vi "new recipe file.vi"() -> ()   [LabVIEW 2018]
uses:
  <vilib>/Utility/file.llb/Read Delimited Spreadsheet (string).vi
panel:
  out "error out 2":errorcluster caption="error out"
  out "error out":errorcluster
  in  "hidden tab":enum32{"Page 1"}(tab)
  out "L pressure":string
  out "L argon flow":string
  out "L rf length step 10":string
  out "L rf length step 9":string
  out "L rf length step 8":string
  out "L rf length step 7":string
  out "L rf length step 6":string
  out "L rf length step 5":string
  out "L rf length step 4":string
  out "L rf length step 3":string
  out "L rf length step 2":string
  out "L rf length step 1":string
  out "L rf power step 10":string
  out "L rf power step 9":string
  out "L rf power step 8":string
  out "L rf power step 7":string
  out "L rf power step 6":string
  out "L rf power step 5":string
  out "L rf power step 4":string
  out "L rf power step 3":string
  out "L rf power step 2":string
  out "L rf power step 1":string
  out "L dc length step 10":string
  out "L dc length step 9":string
  out "L dc length step 8":string
  out "L dc length step 7":string
  out "L dc length step 6":string
  out "L dc length step 5":string
  out "L dc length step 4":string
  out "L dc length step 3":string
  out "L dc length step 2":string
  out "L dc length step 1":string
  out "L dc power step 10":string
  out "L dc power step 9":string
  out "L dc power step 8":string
  out "L dc power step 7":string
  out "L dc power step 6":string
  out "L dc power step 5":string
  out "L dc power step 4":string
  out "L dc power step 3":string
  out "L dc power step 2":string
  out "L dc power step 1":string
  out "L microwave power":string
  out "L chamber selection":string
  out "L single process type selection":string
  out "L tension  value":string
  out "L web speed":string
  out "L web thickness":string
  out "L left init diamater":string
  out "L core diamater":string
  out "L web selection":string
  out "L recipe selection":string
  out "L sbs name":string
  out "L recipe name":string
  out "total length error":bool
  out "left diameter after roll":dbl=8.0
  out "done":bool
  out "L dc step number":string
  out "L rf step number":string
  in  "steplist tab RF":enum32{"Page 1", "Page 2"}(tab)
  in  "rf step watt 1":dbl
  in  "rf step watt 2":dbl
  in  "rf step watt 3":dbl
  in  "rf step watt 4":dbl
  in  "rf step watt 7":dbl
  in  "rf step watt 8":dbl
  in  "rf step watt 5":dbl
  in  "rf step watt 6":dbl
  in  "rf step watt 9":dbl
  in  "rf step watt 10":dbl
  in  "rf step length 1":dbl
  in  "rf step length 2":dbl
  in  "rf step length 3":dbl
  in  "rf step length 4":dbl
  in  "rf step length 5":dbl
  in  "rf step length 6":dbl
  in  "rf step length 7":dbl
  in  "rf step length 8":dbl
  in  "rf step length 9":dbl
  in  "rf step length 10":dbl
  in  "Step Number RF":u16(ring) items=["step 1"=1, "step 2"=2, "step 3"=3, "step 4"=4, "step 5"=5, "step 6"=6, "step 7"=7, "step 8"=8, "step 9"=9, "step 10"=10]
  out "concatenated string":string
  in  "steplist tab DC":enum32{"Page 1", "Page 2"}(tab)
  in  "dc step watt 1":dbl
  in  "dc step watt 2":dbl
  in  "dc step watt 3":dbl
  in  "dc step watt 4":dbl
  in  "dc step watt 5":dbl
  in  "dc step watt 6":dbl
  in  "dc step watt 7":dbl
  in  "dc step watt 8":dbl
  in  "dc step watt 9":dbl
  in  "dc step watt 10":dbl
  in  "dc step length 1":dbl
  in  "dc step length 2":dbl
  in  "dc step length 3":dbl
  in  "dc step length 4":dbl
  in  "dc step length 5":dbl
  in  "dc step length 6":dbl
  in  "dc step length 7":dbl
  in  "dc step length 8":dbl
  in  "dc step length 9":dbl
  in  "dc step length 10":dbl
  in  "Step Number DC":u16(ring) items=["step 1"=1, "step 2"=2, "step 3"=3, "step 4"=4, "step 5"=5, "step 6"=6, "step 7"=7, "step 8"=8, "step 9"=9, "step 10"=10]
  in  "General tab sub vi":enum32{"Page 1"}(tab)
  in  "Pressure set mbar":dbl=0.005 format="%#_1e"
  in  "Ar set sccm":dbl=20.0
  in  "CANCEL":bool
  in  "SAVE":bool
  in  "web-other tab":T1(tab)
  out "total length":dbl=500.0
  in  "tension value":dbl=7.0
  in  "web speed":dbl=250.0
  in  "web thickness":dbl=50.0
  in  "left initial diameter":dbl=94.0
  in  "core diameter":dbl=93.0
  in  "CALCULATE":bool
  in  "Web Selection":u16(ring) items=["web", "other"]
  in  "Recipe Selection":u16(ring) items=["single recipe", "multilayer recipe"]
  in  "Recipe Name":string
  in  "Substrate Material":string
  in  "recipe selection":T2(tab)
  in  "single process selection":enum32{"microwave", "dcsputter", "rfsputter"}(radio)
  in  "single process selection":T3(tab)
  in  "power microwave":dbl
  in  "DC Sputter Chamber Selection":enum32{"chamber II", "chamber III"}(radio)
  in  "power rf":dbl
  in  "web speed ch III ml":dbl=250.0
  in  "web speed ch II ml":dbl=250.0
  in  "LOAD":bool
  in  "password":bool
  in  "password":string
  # "Step List(RF)"
  # "power(watt)"
  # "length(cm)"
  # "Step 1"
  # "Step 2"
  # "Step 3"
  # "Step 4"
  # "Step 5"
  # "Step 6"
  # "Step 7"
  # "Step 8"
  # "Step 9"
  # "Step 10"
  # "Step List(DC)"
  # "power(watt)"
  # "length(cm)"
  # "Step 1"
  # "Step 2"
  # "Step 3"
  # "Step 4"
  # "Step 5"
  # "Step 6"
  # "Step 7"
  # "Step 8"
  # "Step 9"
  # "Step 10"
  # "Recipe Name"
  # "Subsrate Material"
  # "Recipe Selection"
  # "Web Selection"
  # "Argon Flow"
  # "sccm"
  # "Set Pressure"
  # "mbar"
  # "Core Diameter"
  # "mm"
  # "Web Speed"
  # "cm/min"
  # "Left InitialDiameter"
  # "mm"
  # "Tension Value"
  # "N"
  # "µm"
  # "cm"
  # "Web Thickness"
  # "Total Length"
  # "Power"
  # "watt"
  # "Power"
  # "watt"
  # "DCPS PARAMETERS"
  # "Chamber III"
  # "Chamber II"
  # "Web Speed"
  # "cm/min"
  # "Web Speed"
  # "cm/min"
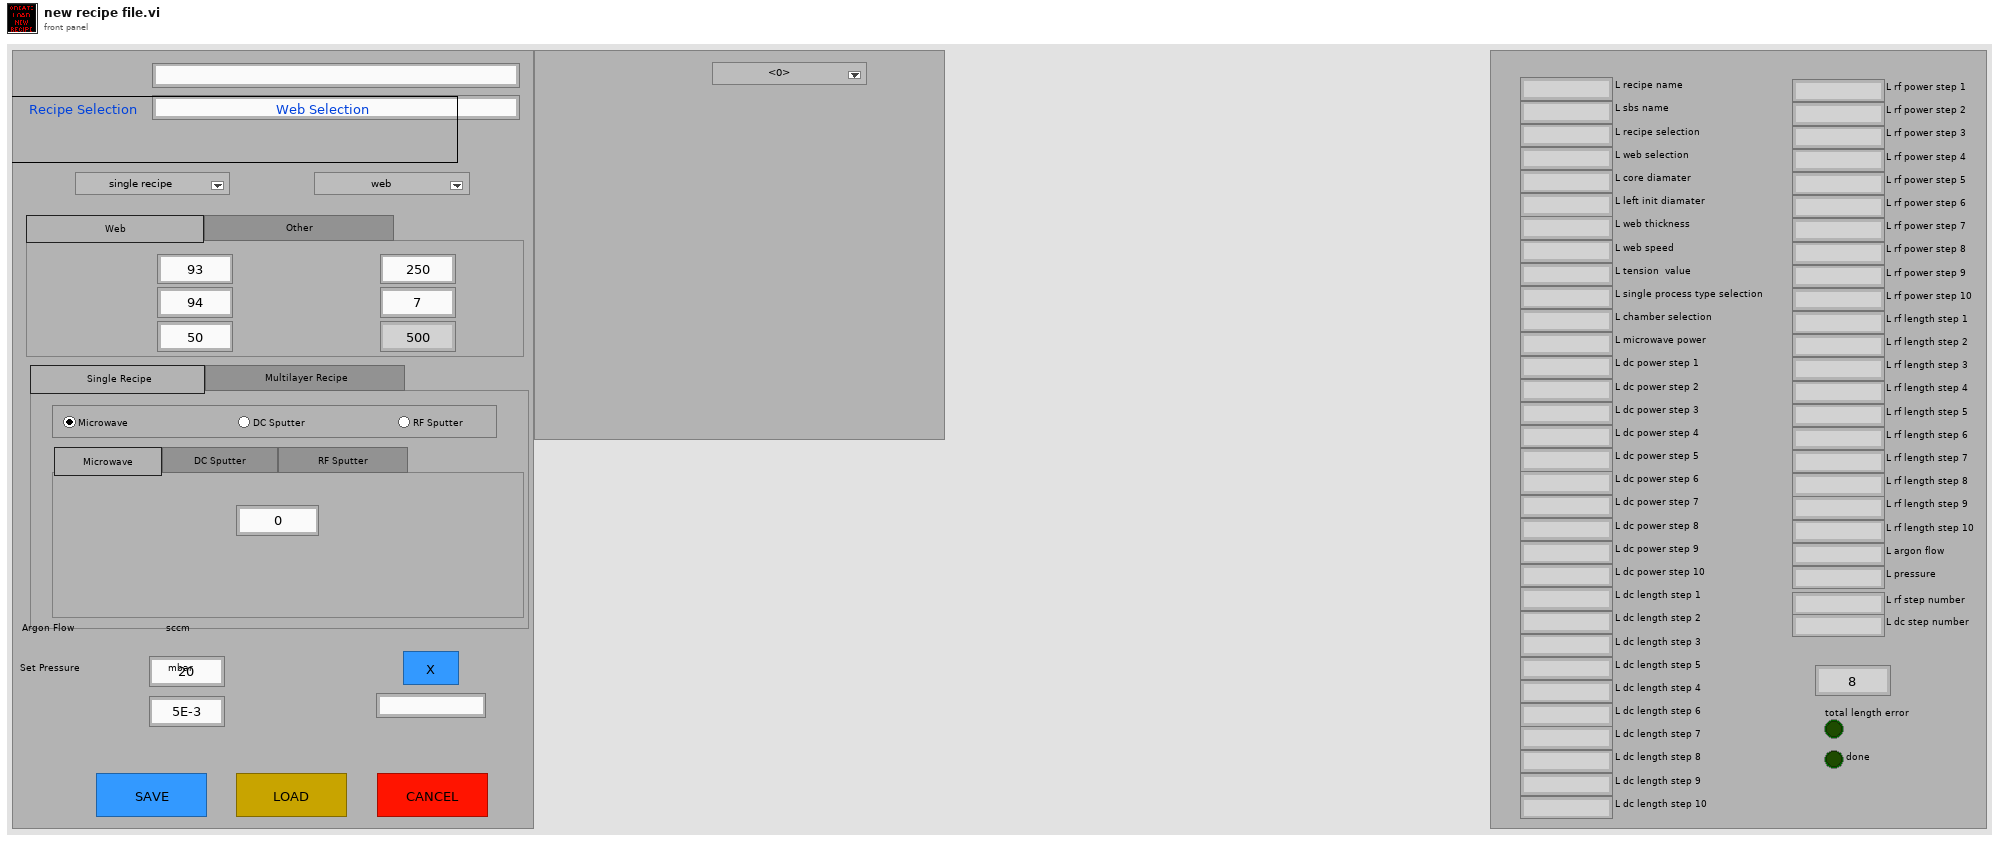
[diagram p1: front panel]
types:
  T1 = enum32{"Web                                                    ", "Other                                                      "}
  T2 = enum32{"Single Recipe                                    ", "Multilayer Recipe                                      "}
  T3 = enum32{"Microwave                ", "DC Sputter                   ", "RF Sputter                         "}
  T4 = enum16{"open", "replace", "create", "open or create", "replace or create", "replace or create with confirmation"}
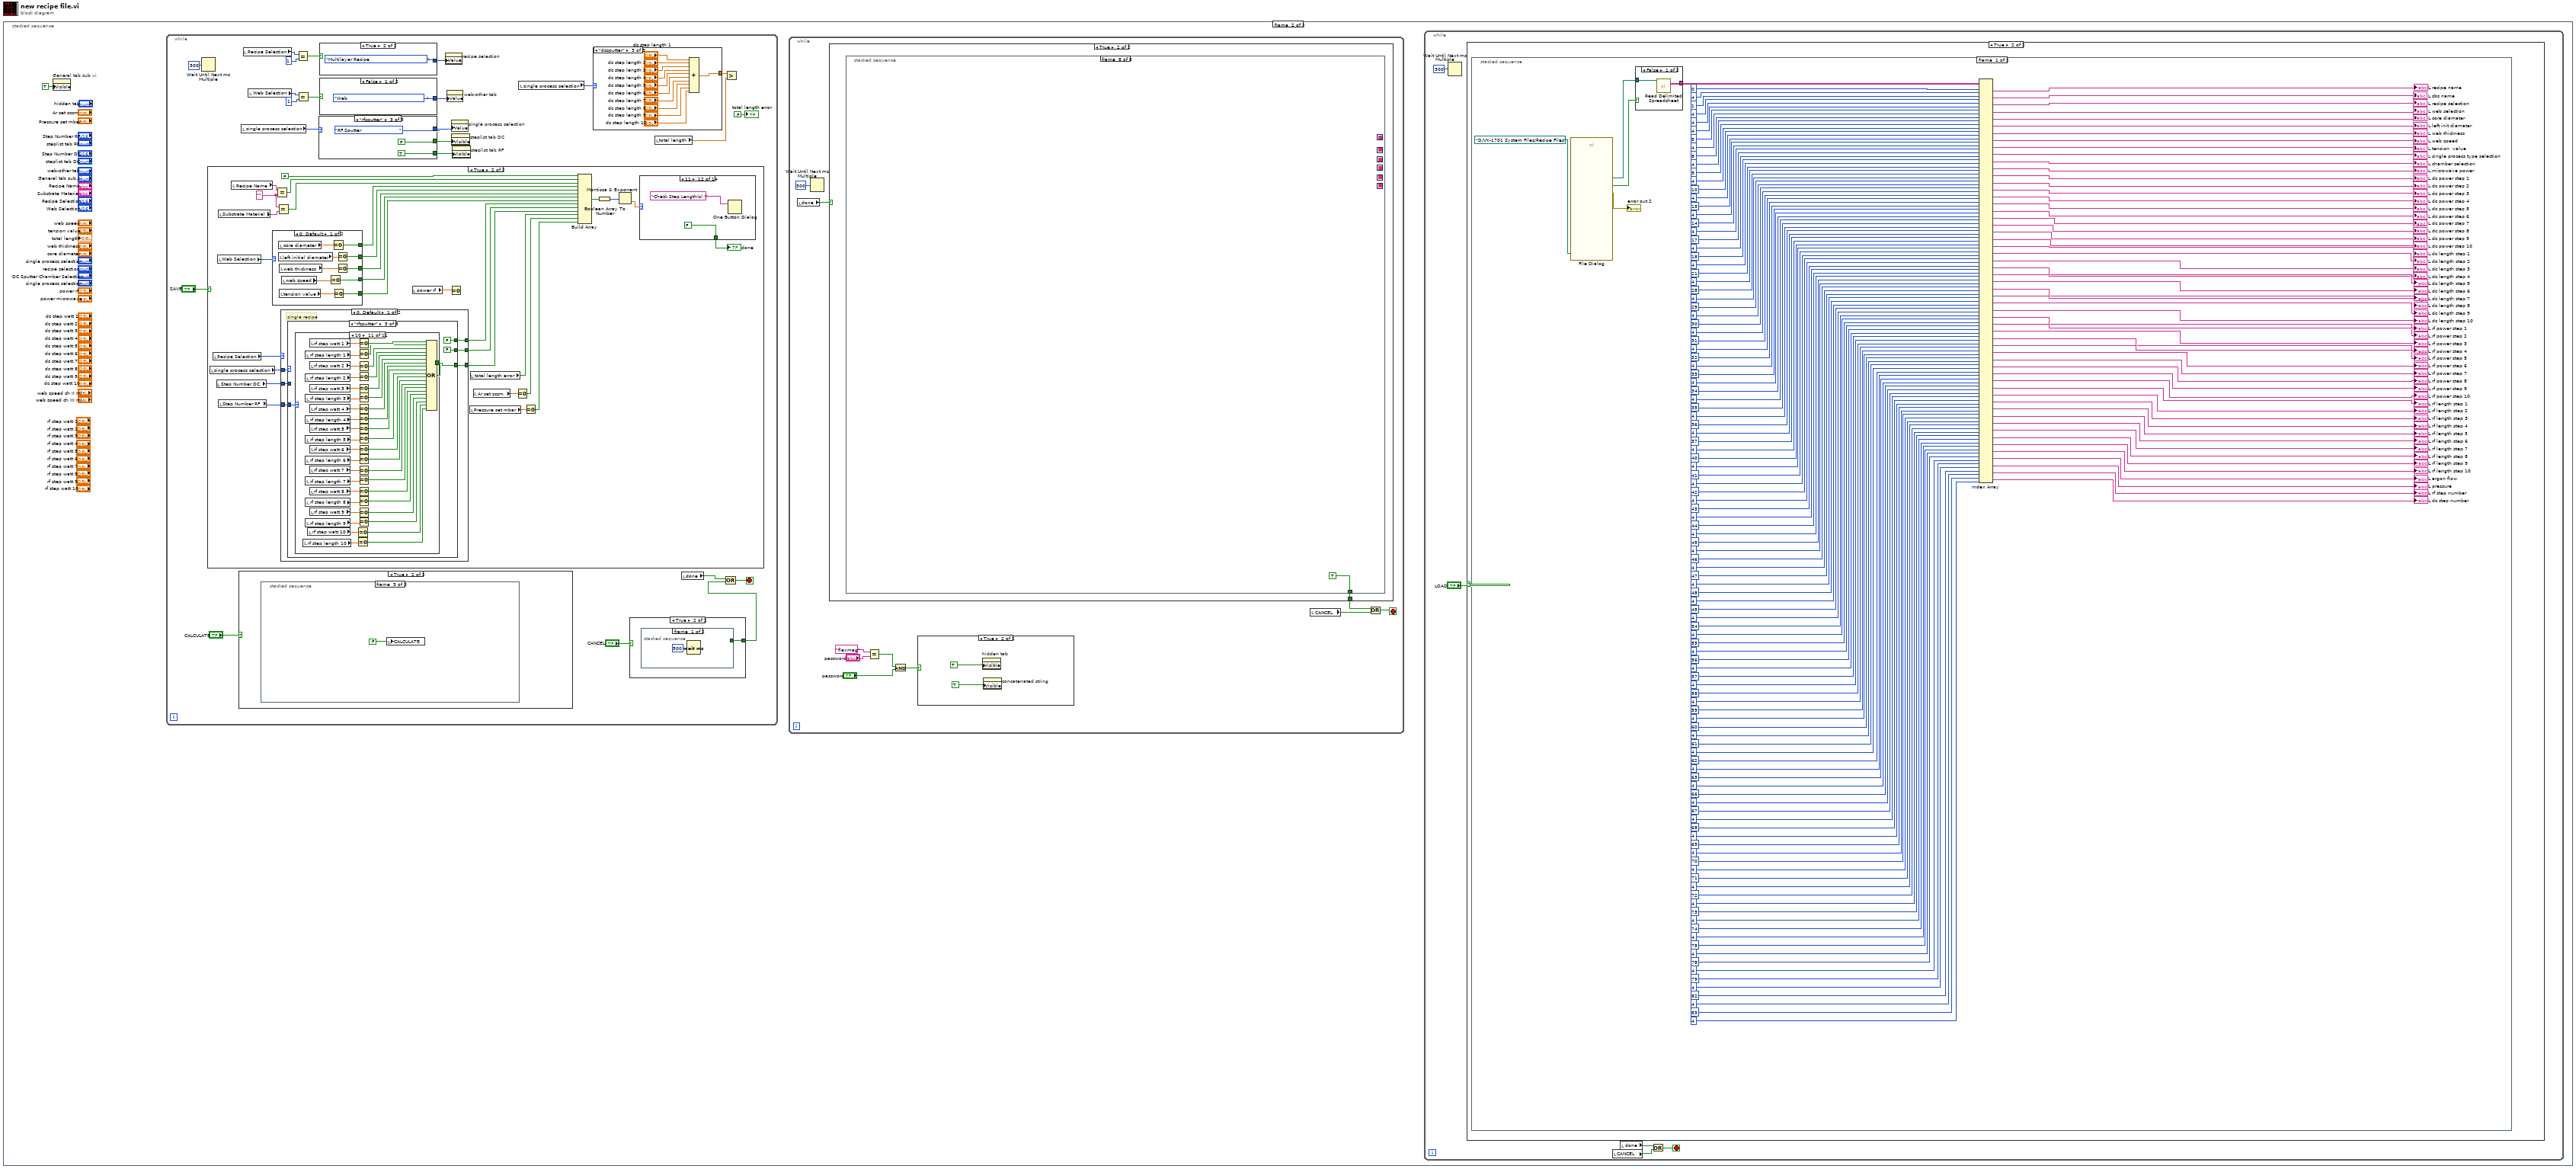
[diagram p0: block diagram]
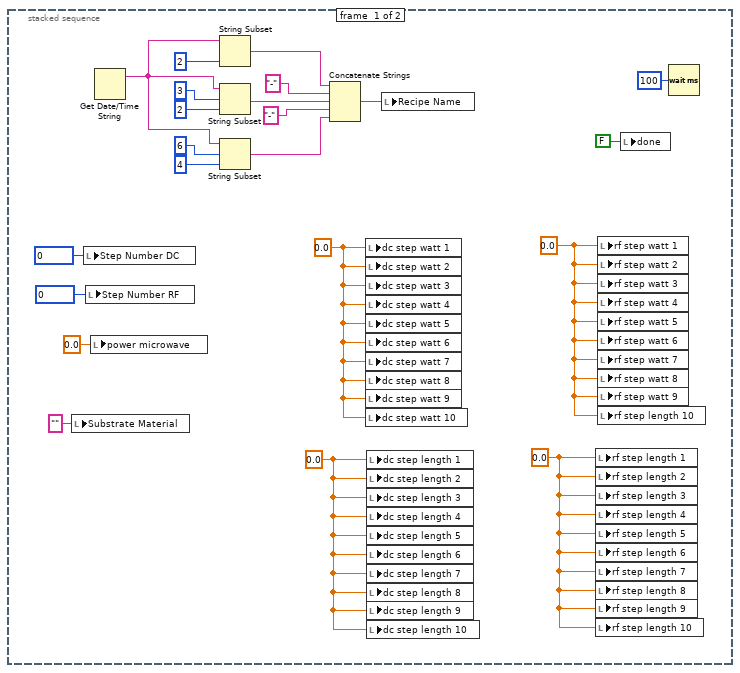
[diagram p2: hidden frame]
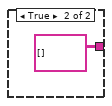
[diagram p4: hidden frame]
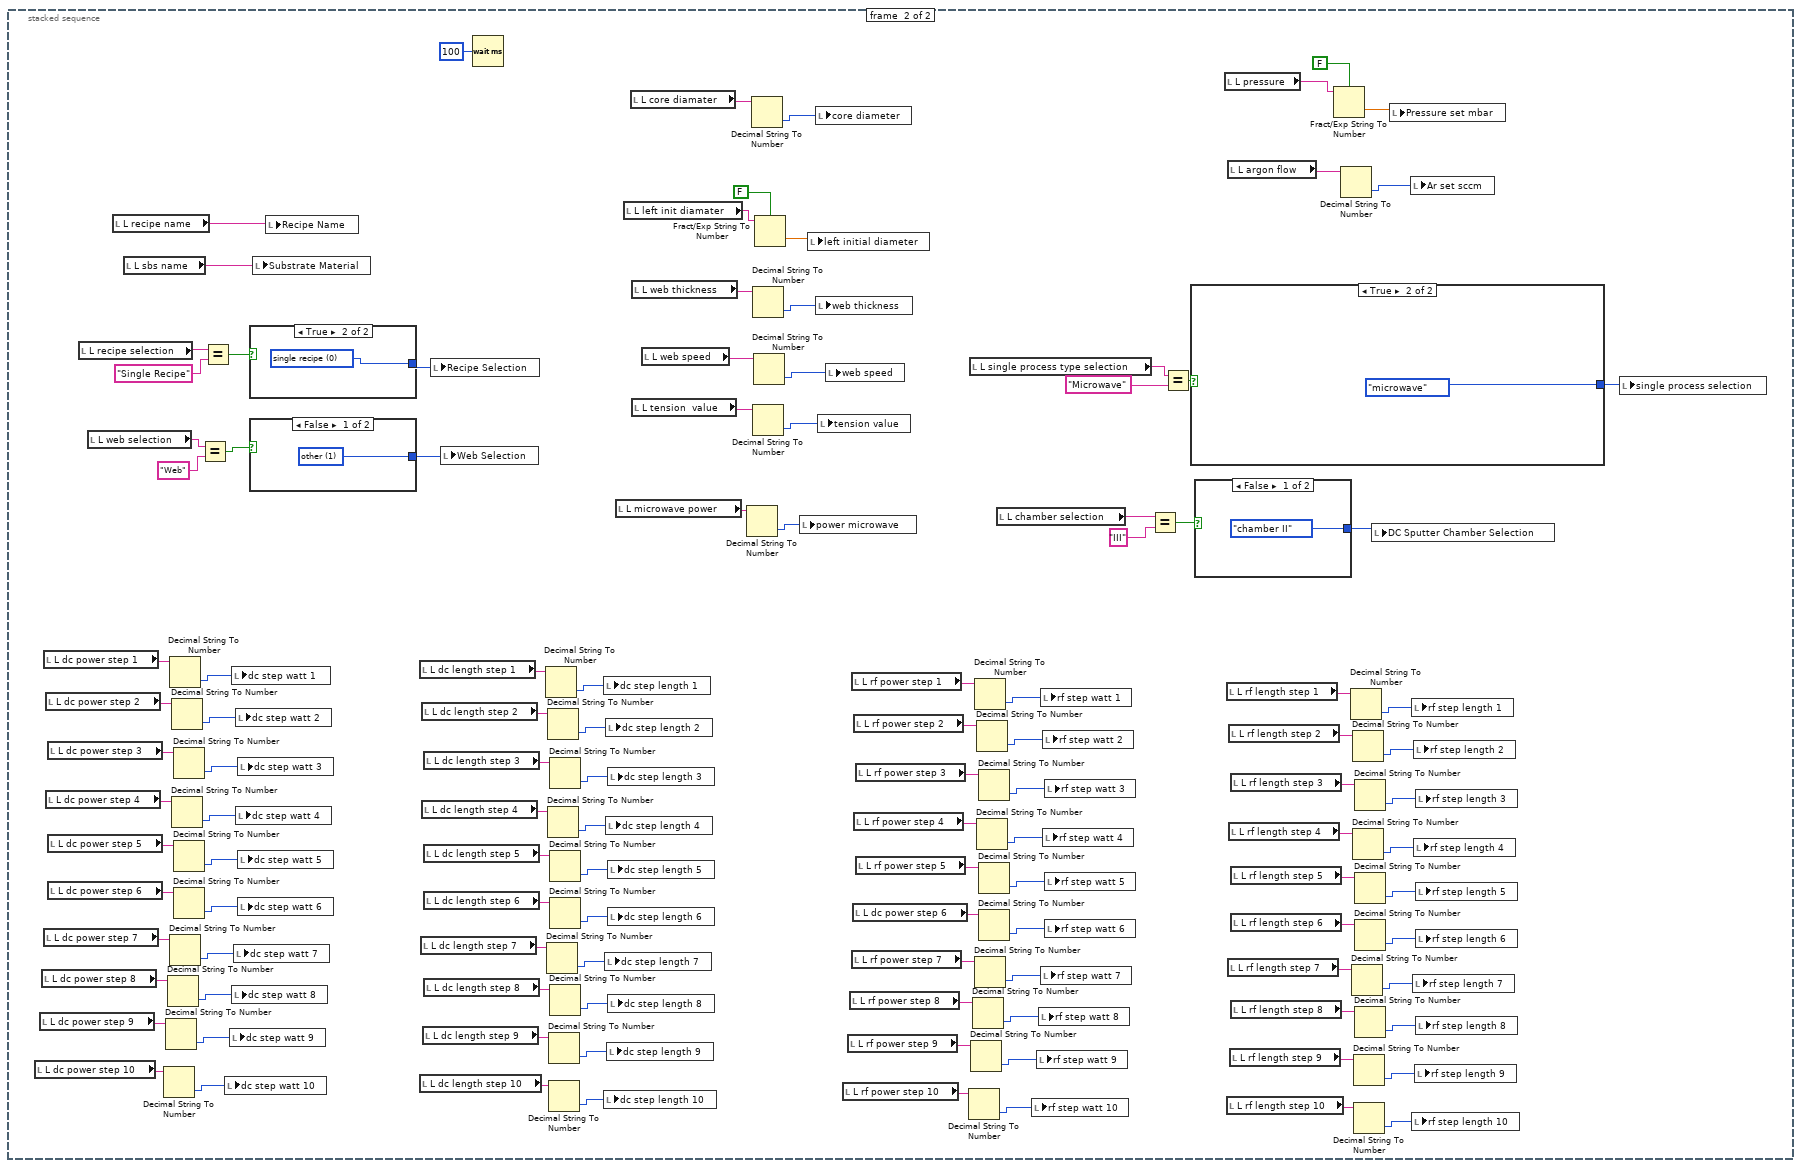
[diagram p5: hidden frame]
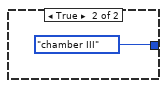
[diagram p6: hidden frame]
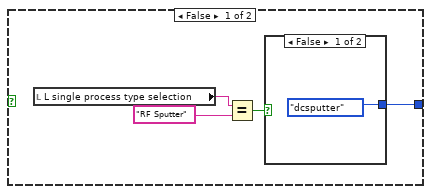
[diagram p7: hidden frame]
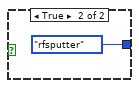
[diagram p8: hidden frame]
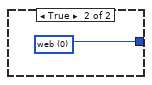
[diagram p9: hidden frame]
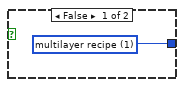
[diagram p10: hidden frame]
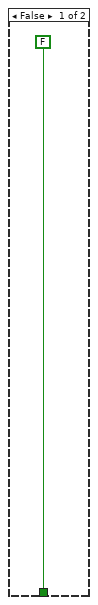
[diagram p12: hidden frame]
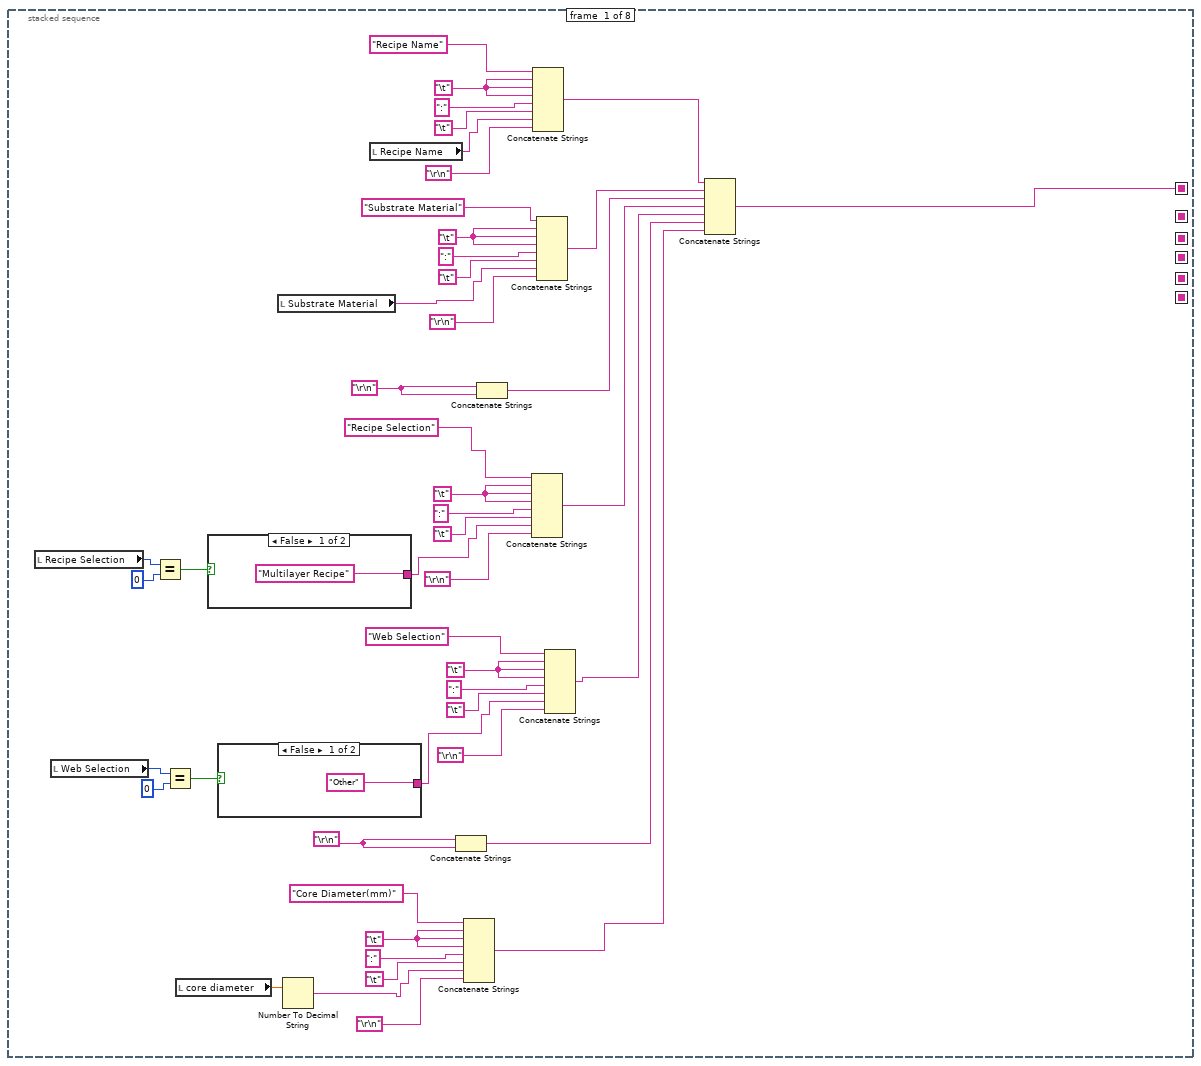
[diagram p13: hidden frame]
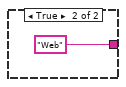
[diagram p14: hidden frame]
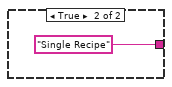
[diagram p15: hidden frame]
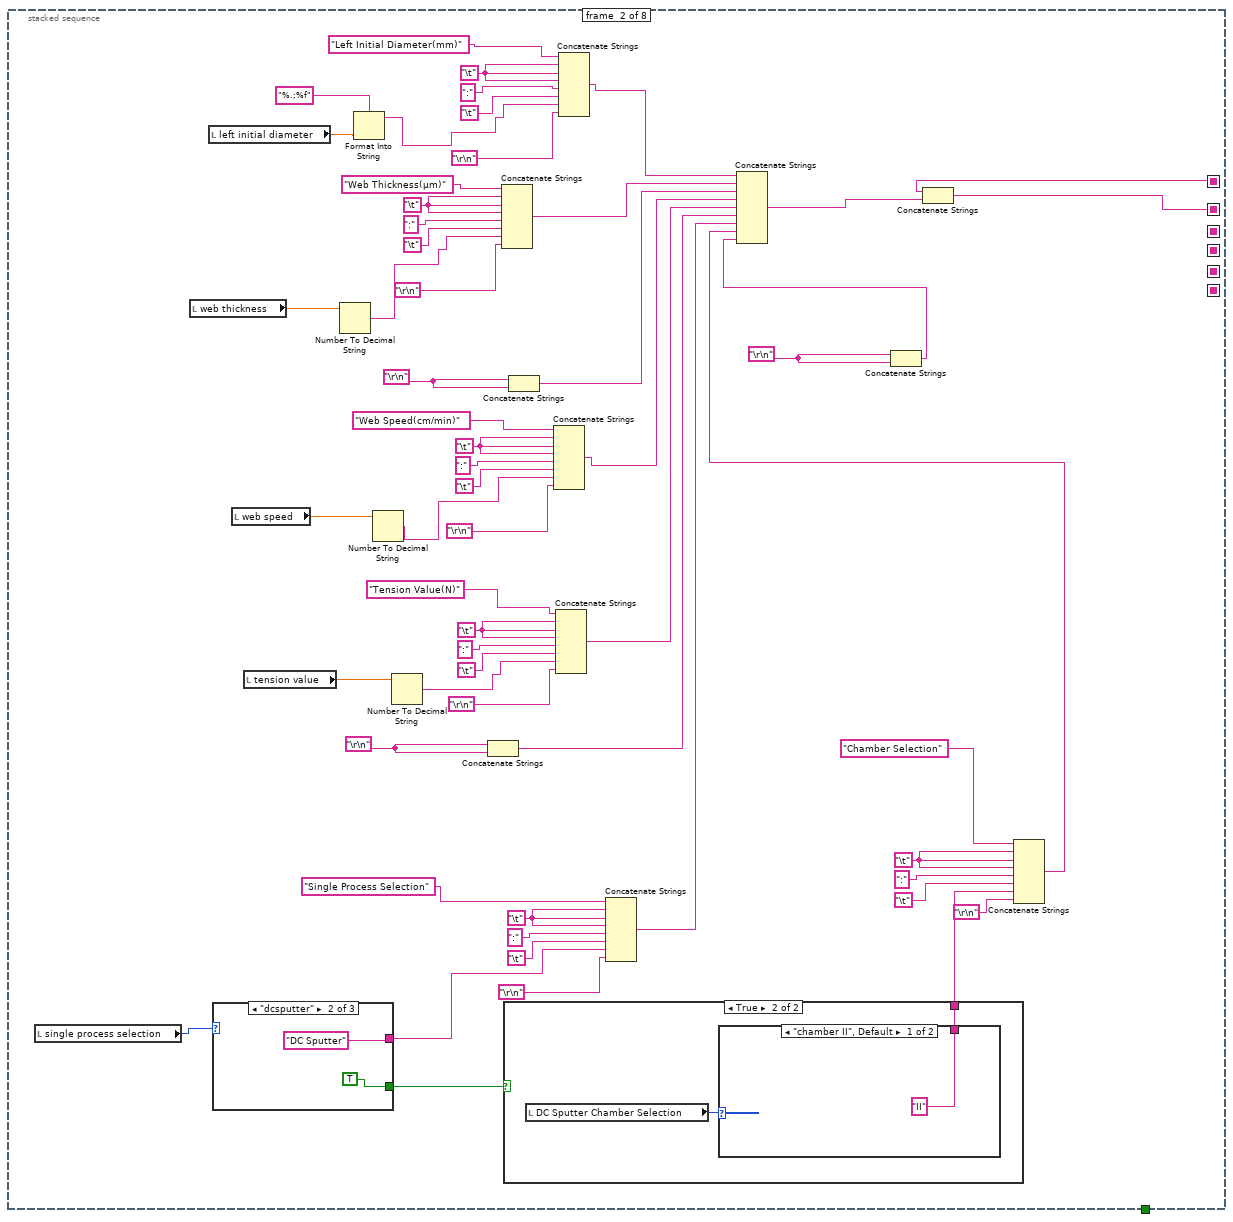
[diagram p16: hidden frame]
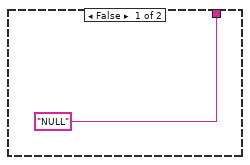
[diagram p17: hidden frame]
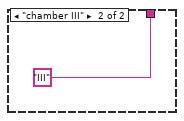
[diagram p18: hidden frame]
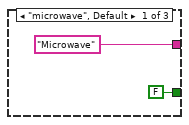
[diagram p19: hidden frame]
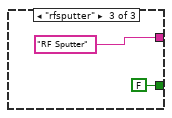
[diagram p20: hidden frame]
diagram:
  n1 = stacked-sequence {
    frame #0 {
      w3 = u16 0 items=["step 1"=1, "step 2"=2, "step 3"=3, "step 4"=4, "step 5"=5, "step 6"=6, "step 7"=7, "step 8"=8, "step 9"=9, "step 10"=10] ("Step Number DC")
      w5 = 0.0 ("dc step watt 1")
      w4 = 0.0 ("dc step watt 1")
      w6 = u16 0 items=["step 1"=1, "step 2"=2, "step 3"=3, "step 4"=4, "step 5"=5, "step 6"=6, "step 7"=7, "step 8"=8, "step 9"=9, "step 10"=10] ("Step Number DC")
      w7 = 0.0 ("dc step watt 1")
      w8 = 0.0 ("dc step watt 1")
      n2 = local write "Substrate Material"("" ("Substrate Material")) -> ()
      n3 = local write "Step Number DC"(w6) -> ()
      n4 = local write "Step Number RF"(w3) -> ()
      n5 = local write "power microwave"(0.0 ("power microwave")) -> ()
      n6 = Get Date/Time String() -> (date string=w16:string)  [unwired: 3 in, 1 out]
      n7 = String Subset(string=w16, length (rest)=2 ("length (rest)")) -> (substring=w17:string)  [unwired: 1 in]
      n8 = String Subset(string=w16, offset (0)=3, length (rest)=2 ("length (rest)")) -> (substring=w18:string)
      n9 = String Subset(string=w16, offset (0)=6, length (rest)=4 ("length (rest)")) -> (substring=w19:string)
      n10 = Concatenate Strings(w17, "-" ("string"), w18, "-" ("string"), w19) -> (w20:string)
      n11 = local write "dc step watt 1"(w8) -> ()
      n12 = local write "dc step watt 2"(w8) -> ()
      n13 = local write "dc step watt 3"(w8) -> ()
      n14 = local write "dc step watt 4"(w8) -> ()
      n15 = local write "dc step watt 5"(w8) -> ()
      n16 = local write "dc step watt 6"(w8) -> ()
      n17 = local write "dc step watt 7"(w8) -> ()
      n18 = local write "dc step watt 8"(w8) -> ()
      n19 = local write "dc step watt 9"(w8) -> ()
      n20 = local write "dc step watt 10"(w8) -> ()
      n21 = local write "dc step length 1"(w7) -> ()
      n22 = local write "dc step length 2"(w7) -> ()
      n23 = local write "dc step length 3"(w7) -> ()
      n24 = local write "dc step length 4"(w7) -> ()
      n25 = local write "dc step length 5"(w7) -> ()
      n26 = local write "dc step length 6"(w7) -> ()
      n27 = local write "dc step length 7"(w7) -> ()
      n28 = local write "dc step length 8"(w7) -> ()
      n29 = local write "dc step length 9"(w7) -> ()
      n30 = local write "dc step length 10"(w7) -> ()
      n31 = local write "Recipe Name"(w20) -> ()
      n32 = local write "rf step length 1"(w5) -> ()
      n33 = local write "rf step length 2"(w5) -> ()
      n34 = local write "rf step length 3"(w5) -> ()
      n35 = local write "rf step length 4"(w5) -> ()
      n36 = local write "rf step length 5"(w5) -> ()
      n37 = local write "rf step length 6"(w5) -> ()
      n38 = local write "rf step length 7"(w5) -> ()
      n39 = local write "rf step length 8"(w5) -> ()
      n40 = local write "rf step length 9"(w5) -> ()
      n41 = local write "rf step length 10"(w5) -> ()
      n42 = local write "rf step watt 1"(w4) -> ()
      n43 = local write "rf step watt 2"(w4) -> ()
      n44 = local write "rf step watt 3"(w4) -> ()
      n45 = local write "rf step watt 4"(w4) -> ()
      n46 = local write "rf step watt 5"(w4) -> ()
      n47 = local write "rf step watt 6"(w4) -> ()
      n48 = local write "rf step watt 7"(w4) -> ()
      n49 = local write "rf step watt 8"(w4) -> ()
      n50 = local write "rf step watt 9"(w4) -> ()
      n51 = local write "rf step length 10"(w4) -> ()
      n52 = local write "done"(FALSE ("done")) -> ()
      n53 = Wait (ms)(milliseconds to wait=u32 100) -> ()  [unwired: 1 out]
    }
    frame #1 {
      n54 = property on="General tab sub vi" class="TabCtl (strict)"("Visible"=TRUE) -> ()  [unwired: 2 in, 2 out]
      n55 = while {
        stop <- w896 stop-if-true
        n56 = Wait Until Next ms Multiple(millisecond multiple=u32 300) -> ()  [unwired: 1 out]
        n57 = case shown="True" "SAVE" {
          frame False {
          }
          frame True {
            w994 = "" ("y")
            n58 = local read "single process selection"() -> (w980:enum32{"microwave", "dcsputter", "rfsputter"})
            n59 = local read "Recipe Selection"() -> (w981:u16)
            n60 = local read "Step Number DC"() -> (w979:u16)
            n61 = local read "Web Selection"() -> (w988:u16)
            n62 = local read "Substrate Material"() -> (w995:string)
            n63 = local read "Step Number RF"() -> (w968:u16)
            n64 = local read "Recipe Name"() -> (w996:string)
            n65 = case shown="0, Default" w988 {
              tunnel: [w1485 w1490] -> w987
              tunnel: [w1484 w1490] -> w986
              tunnel: [w1483 w1490] -> w985
              tunnel: [w1482 w1490] -> w983
              tunnel: [w1480 w1490] -> w984
              frame 0, Default {
                n66 = local read "left initial diameter"() -> (w1488:dbl)
                n67 = local read "core diameter"() -> (w1489:dbl)
                n68 = local read "web thickness"() -> (w1487:dbl)
                n69 = local read "tension value"() -> (w1486:dbl)
                n70 = local read "web speed"() -> (w1481:dbl)
                n71 = Equal To 0?(x=w1481) -> (x = 0?=w1480:bool)
                n72 = Equal To 0?(x=w1489) -> (x = 0?=w1485:bool)
                n73 = Equal To 0?(x=w1486) -> (x = 0?=w1482:bool)
                n74 = Equal To 0?(x=w1488) -> (x = 0?=w1484:bool)
                n75 = Equal To 0?(x=w1487) -> (x = 0?=w1483:bool)
              }
              frame 1 {
                w1490 = FALSE
              }
            }
            n76 = Equal?(x=w996, y=w994) -> (x = y?=w990:bool)
            n77 = Equal?(x=w994, y=w995) -> (x = y?=w989:bool)
            n78 = case shown="0, Default" w981 {
              tunnel: w980 -> [w1002 _]
              tunnel: w979 -> [w1001 _]
              tunnel: [w1000 FALSE] -> w978
              tunnel: [w999 FALSE] -> w977
              tunnel: [w998 FALSE] -> w976
              tunnel: w968 -> [w997 _]
              frame 0, Default {
                # "single recipe"
                n79 = case shown="\"rfsputter\"" w1002 {
                  tunnel: w1001 -> [_ w1010 _]
                  tunnel: [w1005 FALSE FALSE] -> w1000
                  tunnel: [FALSE w1009 FALSE] -> w999
                  tunnel: [FALSE FALSE w1243] -> w998
                  tunnel: w997 -> [_ _ w1242]
                  frame "microwave", Default {
                    n80 = local read "power microwave"() -> (w1006:dbl)
                    n81 = Equal To 0?(x=w1006) -> (x = 0?=w1005:bool)
                  }
                  frame "dcsputter" {
                    n82 = case shown="1" w1010 {
                      tunnel: [FALSE w1012 w1021 w1034 w1051 w1072 w1097 w1126 w1159 w1196 w1237] -> w1009
                      frame 0, Default {
                      }
                      frame 1 {
                        n83 = local read "dc step length 1"() -> (w1015:dbl)
                        n84 = local read "dc step watt 1"() -> (w1016:dbl)
                        n85 = Equal To 0?(x=w1016) -> (x = 0?=w1014:bool)
                        n86 = Equal To 0?(x=w1015) -> (x = 0?=w1013:bool)
                        n87 = Compound Arithmetic op=OR(w1014, w1013) -> (w1012:bool)
                      }
                      frame 2 {
                        n88 = local read "dc step length 1"() -> (w1024:dbl)
                        n89 = local read "dc step length 2"() -> (w1020:dbl)
                        n90 = local read "dc step watt 1"() -> (w1025:dbl)
                        n91 = local read "dc step watt 2"() -> (w1019:dbl)
                        n92 = Equal To 0?(x=w1025) -> (x = 0?=w1023:bool)
                        n93 = Equal To 0?(x=w1019) -> (x = 0?=w1018:bool)
                        n94 = Equal To 0?(x=w1024) -> (x = 0?=w1022:bool)
                        n95 = Equal To 0?(x=w1020) -> (x = 0?=w1017:bool)
                        n96 = Compound Arithmetic op=OR(w1023, w1022, w1018, w1017) -> (w1021:bool)
                      }
                      frame 3 {
                        n97 = local read "dc step length 1"() -> (w1037:dbl)
                        n98 = local read "dc step length 2"() -> (w1033:dbl)
                        n99 = local read "dc step length 3"() -> (w1028:dbl)
                        n100 = local read "dc step watt 1"() -> (w1038:dbl)
                        n101 = local read "dc step watt 2"() -> (w1032:dbl)
                        n102 = local read "dc step watt 3"() -> (w1029:dbl)
                        n103 = Equal To 0?(x=w1038) -> (x = 0?=w1036:bool)
                        n104 = Equal To 0?(x=w1032) -> (x = 0?=w1031:bool)
                        n105 = Equal To 0?(x=w1037) -> (x = 0?=w1035:bool)
                        n106 = Equal To 0?(x=w1029) -> (x = 0?=w1027:bool)
                        n107 = Equal To 0?(x=w1033) -> (x = 0?=w1030:bool)
                        n108 = Equal To 0?(x=w1028) -> (x = 0?=w1026:bool)
                        n109 = Compound Arithmetic op=OR(w1036, w1035, w1031, w1030, w1027, w1026) -> (w1034:bool)
                      }
                      frame 4 {
                        n110 = local read "dc step length 1"() -> (w1054:dbl)
                        n111 = local read "dc step length 4"() -> (w1042:dbl)
                        n112 = local read "dc step length 2"() -> (w1050:dbl)
                        n113 = local read "dc step length 3"() -> (w1045:dbl)
                        n114 = local read "dc step watt 1"() -> (w1055:dbl)
                        n115 = local read "dc step watt 2"() -> (w1049:dbl)
                        n116 = local read "dc step watt 4"() -> (w1041:dbl)
                        n117 = local read "dc step watt 3"() -> (w1046:dbl)
                        n118 = Equal To 0?(x=w1055) -> (x = 0?=w1053:bool)
                        n119 = Equal To 0?(x=w1049) -> (x = 0?=w1048:bool)
                        n120 = Equal To 0?(x=w1041) -> (x = 0?=w1040:bool)
                        n121 = Equal To 0?(x=w1054) -> (x = 0?=w1052:bool)
                        n122 = Equal To 0?(x=w1046) -> (x = 0?=w1044:bool)
                        n123 = Equal To 0?(x=w1042) -> (x = 0?=w1039:bool)
                        n124 = Equal To 0?(x=w1050) -> (x = 0?=w1047:bool)
                        n125 = Equal To 0?(x=w1045) -> (x = 0?=w1043:bool)
                        n126 = Compound Arithmetic op=OR(w1053, w1052, w1048, w1047, w1044, w1043, w1040, w1039) -> (w1051:bool)
                      }
                      frame 5 {
                        n127 = local read "dc step length 5"() -> (w1058:dbl)
                        n128 = local read "dc step length 1"() -> (w1075:dbl)
                        n129 = local read "dc step length 4"() -> (w1063:dbl)
                        n130 = local read "dc step length 2"() -> (w1071:dbl)
                        n131 = local read "dc step length 3"() -> (w1066:dbl)
                        n132 = local read "dc step watt 1"() -> (w1076:dbl)
                        n133 = local read "dc step watt 5"() -> (w1059:dbl)
                        n134 = local read "dc step watt 2"() -> (w1070:dbl)
                        n135 = local read "dc step watt 4"() -> (w1062:dbl)
                        n136 = local read "dc step watt 3"() -> (w1067:dbl)
                        n137 = Equal To 0?(x=w1059) -> (x = 0?=w1057:bool)
                        n138 = Equal To 0?(x=w1076) -> (x = 0?=w1074:bool)
                        n139 = Equal To 0?(x=w1058) -> (x = 0?=w1056:bool)
                        n140 = Equal To 0?(x=w1070) -> (x = 0?=w1069:bool)
                        n141 = Equal To 0?(x=w1062) -> (x = 0?=w1061:bool)
                        n142 = Equal To 0?(x=w1075) -> (x = 0?=w1073:bool)
                        n143 = Equal To 0?(x=w1067) -> (x = 0?=w1065:bool)
                        n144 = Equal To 0?(x=w1063) -> (x = 0?=w1060:bool)
                        n145 = Equal To 0?(x=w1071) -> (x = 0?=w1068:bool)
                        n146 = Equal To 0?(x=w1066) -> (x = 0?=w1064:bool)
                        n147 = Compound Arithmetic op=OR(w1074, w1073, w1069, w1068, w1065, w1064, w1061, w1060, w1057, w1056) -> (w1072:bool)
                      }
                      frame 6 {
                        n148 = local read "dc step length 6"() -> (w1080:dbl)
                        n149 = local read "dc step length 5"() -> (w1083:dbl)
                        n150 = local read "dc step length 1"() -> (w1100:dbl)
                        n151 = local read "dc step length 4"() -> (w1088:dbl)
                        n152 = local read "dc step length 2"() -> (w1096:dbl)
                        n153 = local read "dc step length 3"() -> (w1091:dbl)
                        n154 = local read "dc step watt 6"() -> (w1079:dbl)
                        n155 = local read "dc step watt 1"() -> (w1101:dbl)
                        n156 = local read "dc step watt 5"() -> (w1084:dbl)
                        n157 = local read "dc step watt 2"() -> (w1095:dbl)
                        n158 = local read "dc step watt 4"() -> (w1087:dbl)
                        n159 = local read "dc step watt 3"() -> (w1092:dbl)
                        n160 = Equal To 0?(x=w1079) -> (x = 0?=w1078:bool)
                        n161 = Equal To 0?(x=w1080) -> (x = 0?=w1077:bool)
                        n162 = Equal To 0?(x=w1084) -> (x = 0?=w1082:bool)
                        n163 = Equal To 0?(x=w1101) -> (x = 0?=w1099:bool)
                        n164 = Equal To 0?(x=w1083) -> (x = 0?=w1081:bool)
                        n165 = Equal To 0?(x=w1095) -> (x = 0?=w1094:bool)
                        n166 = Equal To 0?(x=w1087) -> (x = 0?=w1086:bool)
                        n167 = Equal To 0?(x=w1100) -> (x = 0?=w1098:bool)
                        n168 = Equal To 0?(x=w1092) -> (x = 0?=w1090:bool)
                        n169 = Equal To 0?(x=w1088) -> (x = 0?=w1085:bool)
                        n170 = Equal To 0?(x=w1096) -> (x = 0?=w1093:bool)
                        n171 = Equal To 0?(x=w1091) -> (x = 0?=w1089:bool)
                        n172 = Compound Arithmetic op=OR(w1099, w1098, w1094, w1093, w1090, w1089, w1086, w1085, w1082, w1081, w1078, w1077) -> (w1097:bool)
                      }
                      frame 7 {
                        n173 = local read "dc step length 6"() -> (w1109:dbl)
                        n174 = local read "dc step length 7"() -> (w1104:dbl)
                        n175 = local read "dc step length 5"() -> (w1112:dbl)
                        n176 = local read "dc step length 1"() -> (w1129:dbl)
                        n177 = local read "dc step length 4"() -> (w1117:dbl)
                        n178 = local read "dc step length 2"() -> (w1125:dbl)
                        n179 = local read "dc step length 3"() -> (w1120:dbl)
                        n180 = local read "dc step watt 6"() -> (w1108:dbl)
                        n181 = local read "dc step watt 7"() -> (w1105:dbl)
                        n182 = local read "dc step watt 1"() -> (w1130:dbl)
                        n183 = local read "dc step watt 5"() -> (w1113:dbl)
                        n184 = local read "dc step watt 2"() -> (w1124:dbl)
                        n185 = local read "dc step watt 4"() -> (w1116:dbl)
                        n186 = local read "dc step watt 3"() -> (w1121:dbl)
                        n187 = Equal To 0?(x=w1108) -> (x = 0?=w1107:bool)
                        n188 = Equal To 0?(x=w1105) -> (x = 0?=w1103:bool)
                        n189 = Equal To 0?(x=w1109) -> (x = 0?=w1106:bool)
                        n190 = Equal To 0?(x=w1104) -> (x = 0?=w1102:bool)
                        n191 = Equal To 0?(x=w1113) -> (x = 0?=w1111:bool)
                        n192 = Equal To 0?(x=w1130) -> (x = 0?=w1128:bool)
                        n193 = Equal To 0?(x=w1112) -> (x = 0?=w1110:bool)
                        n194 = Equal To 0?(x=w1124) -> (x = 0?=w1123:bool)
                        n195 = Equal To 0?(x=w1116) -> (x = 0?=w1115:bool)
                        n196 = Equal To 0?(x=w1129) -> (x = 0?=w1127:bool)
                        n197 = Equal To 0?(x=w1121) -> (x = 0?=w1119:bool)
                        n198 = Equal To 0?(x=w1117) -> (x = 0?=w1114:bool)
                        n199 = Equal To 0?(x=w1125) -> (x = 0?=w1122:bool)
                        n200 = Equal To 0?(x=w1120) -> (x = 0?=w1118:bool)
                        n201 = Compound Arithmetic op=OR(w1128, w1127, w1123, w1122, w1119, w1118, w1115, w1114, w1111, w1110, w1107, w1106, w1103, w1102) -> (w1126:bool)
                      }
                      frame 8 {
                        n202 = local read "dc step length 6"() -> (w1142:dbl)
                        n203 = local read "dc step length 7"() -> (w1137:dbl)
                        n204 = local read "dc step length 8"() -> (w1134:dbl)
                        n205 = local read "dc step length 5"() -> (w1145:dbl)
                        n206 = local read "dc step length 1"() -> (w1162:dbl)
                        n207 = local read "dc step length 4"() -> (w1150:dbl)
                        n208 = local read "dc step length 2"() -> (w1158:dbl)
                        n209 = local read "dc step length 3"() -> (w1153:dbl)
                        n210 = local read "dc step watt 6"() -> (w1141:dbl)
                        n211 = local read "dc step watt 7"() -> (w1138:dbl)
                        n212 = local read "dc step watt 8"() -> (w1133:dbl)
                        n213 = local read "dc step watt 1"() -> (w1163:dbl)
                        n214 = local read "dc step watt 5"() -> (w1146:dbl)
                        n215 = local read "dc step watt 2"() -> (w1157:dbl)
                        n216 = local read "dc step watt 4"() -> (w1149:dbl)
                        n217 = local read "dc step watt 3"() -> (w1154:dbl)
                        n218 = Equal To 0?(x=w1141) -> (x = 0?=w1140:bool)
                        n219 = Equal To 0?(x=w1138) -> (x = 0?=w1136:bool)
                        n220 = Equal To 0?(x=w1142) -> (x = 0?=w1139:bool)
                        n221 = Equal To 0?(x=w1137) -> (x = 0?=w1135:bool)
                        n222 = Equal To 0?(x=w1133) -> (x = 0?=w1132:bool)
                        n223 = Equal To 0?(x=w1146) -> (x = 0?=w1144:bool)
                        n224 = Equal To 0?(x=w1134) -> (x = 0?=w1131:bool)
                        n225 = Equal To 0?(x=w1163) -> (x = 0?=w1161:bool)
                        n226 = Equal To 0?(x=w1145) -> (x = 0?=w1143:bool)
                        n227 = Equal To 0?(x=w1157) -> (x = 0?=w1156:bool)
                        n228 = Equal To 0?(x=w1149) -> (x = 0?=w1148:bool)
                        n229 = Equal To 0?(x=w1162) -> (x = 0?=w1160:bool)
                        n230 = Equal To 0?(x=w1154) -> (x = 0?=w1152:bool)
                        n231 = Equal To 0?(x=w1150) -> (x = 0?=w1147:bool)
                        n232 = Equal To 0?(x=w1158) -> (x = 0?=w1155:bool)
                        n233 = Equal To 0?(x=w1153) -> (x = 0?=w1151:bool)
                        n234 = Compound Arithmetic op=OR(w1161, w1160, w1156, w1155, w1152, w1151, w1148, w1147, w1144, w1143, w1140, w1139, w1136, w1135, w1132, w1131) -> (w1159:bool)
                      }
                      frame 9 {
                        n235 = local read "dc step length 1"() -> (w1199:dbl)
                        n236 = local read "dc step length 2"() -> (w1195:dbl)
                        n237 = local read "dc step length 3"() -> (w1190:dbl)
                        n238 = local read "dc step length 4"() -> (w1187:dbl)
                        n239 = local read "dc step length 5"() -> (w1182:dbl)
                        n240 = local read "dc step length 6"() -> (w1179:dbl)
                        n241 = local read "dc step length 7"() -> (w1174:dbl)
                        n242 = local read "dc step length 8"() -> (w1171:dbl)
                        n243 = local read "dc step length 9"() -> (w1166:dbl)
                        n244 = local read "dc step watt 1"() -> (w1200:dbl)
                        n245 = local read "dc step watt 2"() -> (w1194:dbl)
                        n246 = local read "dc step watt 3"() -> (w1191:dbl)
                        n247 = local read "dc step watt 4"() -> (w1186:dbl)
                        n248 = local read "dc step watt 5"() -> (w1183:dbl)
                        n249 = local read "dc step watt 6"() -> (w1178:dbl)
                        n250 = local read "dc step watt 7"() -> (w1175:dbl)
                        n251 = local read "dc step watt 8"() -> (w1170:dbl)
                        n252 = local read "dc step watt 9"() -> (w1167:dbl)
                        n253 = Equal To 0?(x=w1178) -> (x = 0?=w1177:bool)
                        n254 = Equal To 0?(x=w1175) -> (x = 0?=w1173:bool)
                        n255 = Equal To 0?(x=w1179) -> (x = 0?=w1176:bool)
                        n256 = Equal To 0?(x=w1174) -> (x = 0?=w1172:bool)
                        n257 = Equal To 0?(x=w1170) -> (x = 0?=w1169:bool)
                        n258 = Equal To 0?(x=w1183) -> (x = 0?=w1181:bool)
                        n259 = Equal To 0?(x=w1171) -> (x = 0?=w1168:bool)
                        n260 = Equal To 0?(x=w1200) -> (x = 0?=w1198:bool)
                        n261 = Equal To 0?(x=w1182) -> (x = 0?=w1180:bool)
                        n262 = Equal To 0?(x=w1194) -> (x = 0?=w1193:bool)
                        n263 = Equal To 0?(x=w1186) -> (x = 0?=w1185:bool)
                        n264 = Equal To 0?(x=w1167) -> (x = 0?=w1165:bool)
                        n265 = Equal To 0?(x=w1199) -> (x = 0?=w1197:bool)
                        n266 = Equal To 0?(x=w1191) -> (x = 0?=w1189:bool)
                        n267 = Equal To 0?(x=w1187) -> (x = 0?=w1184:bool)
                        n268 = Equal To 0?(x=w1195) -> (x = 0?=w1192:bool)
                        n269 = Equal To 0?(x=w1190) -> (x = 0?=w1188:bool)
                        n270 = Equal To 0?(x=w1166) -> (x = 0?=w1164:bool)
                        n271 = Compound Arithmetic op=OR(w1198, w1197, w1193, w1192, w1189, w1188, w1185, w1184, w1181, w1180, w1177, w1176, w1173, w1172, w1169, w1168, w1165, w1164) -> (w1196:bool)
                      }
                      frame 10 {
                        n272 = local read "dc step length 10"() -> (w1204:dbl)
                        n273 = local read "dc step length 1"() -> (w1240:dbl)
                        n274 = local read "dc step length 2"() -> (w1236:dbl)
                        n275 = local read "dc step length 3"() -> (w1231:dbl)
                        n276 = local read "dc step length 4"() -> (w1228:dbl)
                        n277 = local read "dc step length 5"() -> (w1223:dbl)
                        n278 = local read "dc step length 6"() -> (w1220:dbl)
                        n279 = local read "dc step length 7"() -> (w1215:dbl)
                        n280 = local read "dc step length 8"() -> (w1212:dbl)
                        n281 = local read "dc step length 9"() -> (w1207:dbl)
                        n282 = local read "dc step watt 10"() -> (w1203:dbl)
                        n283 = local read "dc step watt 1"() -> (w1241:dbl)
                        n284 = local read "dc step watt 2"() -> (w1235:dbl)
                        n285 = local read "dc step watt 3"() -> (w1232:dbl)
                        n286 = local read "dc step watt 4"() -> (w1227:dbl)
                        n287 = local read "dc step watt 5"() -> (w1224:dbl)
                        n288 = local read "dc step watt 6"() -> (w1219:dbl)
                        n289 = local read "dc step watt 7"() -> (w1216:dbl)
                        n290 = local read "dc step watt 8"() -> (w1211:dbl)
                        n291 = local read "dc step watt 9"() -> (w1208:dbl)
                        n292 = Equal To 0?(x=w1241) -> (x = 0?=w1239:bool)
                        n293 = Equal To 0?(x=w1240) -> (x = 0?=w1238:bool)
                        n294 = Equal To 0?(x=w1235) -> (x = 0?=w1234:bool)
                        n295 = Equal To 0?(x=w1236) -> (x = 0?=w1233:bool)
                        n296 = Equal To 0?(x=w1232) -> (x = 0?=w1230:bool)
                        n297 = Equal To 0?(x=w1231) -> (x = 0?=w1229:bool)
                        n298 = Equal To 0?(x=w1227) -> (x = 0?=w1226:bool)
                        n299 = Equal To 0?(x=w1228) -> (x = 0?=w1225:bool)
                        n300 = Equal To 0?(x=w1224) -> (x = 0?=w1222:bool)
                        n301 = Equal To 0?(x=w1223) -> (x = 0?=w1221:bool)
                        n302 = Equal To 0?(x=w1219) -> (x = 0?=w1218:bool)
                        n303 = Equal To 0?(x=w1220) -> (x = 0?=w1217:bool)
                        n304 = Equal To 0?(x=w1216) -> (x = 0?=w1214:bool)
                        n305 = Equal To 0?(x=w1215) -> (x = 0?=w1213:bool)
                        n306 = Equal To 0?(x=w1211) -> (x = 0?=w1210:bool)
                        n307 = Equal To 0?(x=w1212) -> (x = 0?=w1209:bool)
                        n308 = Equal To 0?(x=w1208) -> (x = 0?=w1206:bool)
                        n309 = Equal To 0?(x=w1207) -> (x = 0?=w1205:bool)
                        n310 = Equal To 0?(x=w1203) -> (x = 0?=w1202:bool)
                        n311 = Equal To 0?(x=w1204) -> (x = 0?=w1201:bool)
                        n312 = Compound Arithmetic op=OR(w1239, w1238, w1234, w1233, w1230, w1229, w1226, w1225, w1222, w1221, w1218, w1217, w1214, w1213, w1210, w1209, w1206, w1205, w1202, w1201) -> (w1237:bool)
                      }
                    }
                  }
                  frame "rfsputter" {
                    n313 = case shown="10" w1242 {
                      tunnel: [FALSE w1247 w1256 w1269 w1286 w1307 w1332 w1361 w1394 w1431 w1472] -> w1243
                      frame 0, Default {
                      }
                      frame 1 {
                        n314 = local read "rf step length 1"() -> (w1250:dbl)
                        n315 = local read "rf step watt 1"() -> (w1251:dbl)
                        n316 = Equal To 0?(x=w1251) -> (x = 0?=w1249:bool)
                        n317 = Equal To 0?(x=w1250) -> (x = 0?=w1248:bool)
                        n318 = Compound Arithmetic op=OR(w1249, w1248) -> (w1247:bool)
                      }
                      frame 2 {
                        n319 = local read "rf step length 1"() -> (w1259:dbl)
                        n320 = local read "rf step length 2"() -> (w1255:dbl)
                        n321 = local read "rf step watt 1"() -> (w1260:dbl)
                        n322 = local read "rf step watt 2"() -> (w1254:dbl)
                        n323 = Equal To 0?(x=w1260) -> (x = 0?=w1258:bool)
                        n324 = Equal To 0?(x=w1254) -> (x = 0?=w1253:bool)
                        n325 = Equal To 0?(x=w1259) -> (x = 0?=w1257:bool)
                        n326 = Equal To 0?(x=w1255) -> (x = 0?=w1252:bool)
                        n327 = Compound Arithmetic op=OR(w1258, w1257, w1253, w1252) -> (w1256:bool)
                      }
                      frame 3 {
                        n328 = local read "rf step length 1"() -> (w1272:dbl)
                        n329 = local read "rf step length 2"() -> (w1268:dbl)
                        n330 = local read "rf step length 3"() -> (w1263:dbl)
                        n331 = local read "rf step watt 1"() -> (w1273:dbl)
                        n332 = local read "rf step watt 2"() -> (w1267:dbl)
                        n333 = local read "rf step watt 3"() -> (w1264:dbl)
                        n334 = Equal To 0?(x=w1273) -> (x = 0?=w1271:bool)
                        n335 = Equal To 0?(x=w1267) -> (x = 0?=w1266:bool)
                        n336 = Equal To 0?(x=w1272) -> (x = 0?=w1270:bool)
                        n337 = Equal To 0?(x=w1264) -> (x = 0?=w1262:bool)
                        n338 = Equal To 0?(x=w1268) -> (x = 0?=w1265:bool)
                        n339 = Equal To 0?(x=w1263) -> (x = 0?=w1261:bool)
                        n340 = Compound Arithmetic op=OR(w1271, w1270, w1266, w1265, w1262, w1261) -> (w1269:bool)
                      }
                      frame 4 {
                        n341 = local read "rf step length 1"() -> (w1289:dbl)
                        n342 = local read "rf step length 4"() -> (w1277:dbl)
                        n343 = local read "rf step length 2"() -> (w1285:dbl)
                        n344 = local read "rf step length 3"() -> (w1280:dbl)
                        n345 = local read "rf step watt 1"() -> (w1290:dbl)
                        n346 = local read "rf step watt 2"() -> (w1284:dbl)
                        n347 = local read "rf step watt 4"() -> (w1276:dbl)
                        n348 = local read "rf step watt 3"() -> (w1281:dbl)
                        n349 = Equal To 0?(x=w1290) -> (x = 0?=w1288:bool)
                        n350 = Equal To 0?(x=w1284) -> (x = 0?=w1283:bool)
                        n351 = Equal To 0?(x=w1276) -> (x = 0?=w1275:bool)
                        n352 = Equal To 0?(x=w1289) -> (x = 0?=w1287:bool)
                        n353 = Equal To 0?(x=w1281) -> (x = 0?=w1279:bool)
                        n354 = Equal To 0?(x=w1277) -> (x = 0?=w1274:bool)
                        n355 = Equal To 0?(x=w1285) -> (x = 0?=w1282:bool)
                        n356 = Equal To 0?(x=w1280) -> (x = 0?=w1278:bool)
                        n357 = Compound Arithmetic op=OR(w1288, w1287, w1283, w1282, w1279, w1278, w1275, w1274) -> (w1286:bool)
                      }
                      frame 5 {
                        n358 = local read "rf step length 1"() -> (w1310:dbl)
                        n359 = local read "rf step length 2"() -> (w1306:dbl)
                        n360 = local read "rf step length 3"() -> (w1301:dbl)
                        n361 = local read "rf step length 4"() -> (w1298:dbl)
                        n362 = local read "rf step length 5"() -> (w1293:dbl)
                        n363 = local read "rf step watt 1"() -> (w1311:dbl)
                        n364 = local read "rf step watt 2"() -> (w1305:dbl)
                        n365 = local read "rf step watt 3"() -> (w1302:dbl)
                        n366 = local read "rf step watt 4"() -> (w1297:dbl)
                        n367 = local read "rf step watt 5"() -> (w1294:dbl)
                        n368 = Equal To 0?(x=w1311) -> (x = 0?=w1309:bool)
                        n369 = Equal To 0?(x=w1310) -> (x = 0?=w1308:bool)
                        n370 = Equal To 0?(x=w1305) -> (x = 0?=w1304:bool)
                        n371 = Equal To 0?(x=w1306) -> (x = 0?=w1303:bool)
                        n372 = Equal To 0?(x=w1302) -> (x = 0?=w1300:bool)
                        n373 = Equal To 0?(x=w1301) -> (x = 0?=w1299:bool)
                        n374 = Equal To 0?(x=w1297) -> (x = 0?=w1296:bool)
                        n375 = Equal To 0?(x=w1298) -> (x = 0?=w1295:bool)
                        n376 = Equal To 0?(x=w1294) -> (x = 0?=w1292:bool)
                        n377 = Equal To 0?(x=w1293) -> (x = 0?=w1291:bool)
                        n378 = Compound Arithmetic op=OR(w1309, w1308, w1304, w1303, w1300, w1299, w1296, w1295, w1292, w1291) -> (w1307:bool)
                      }
                      frame 6 {
                        n379 = local read "rf step length 3"() -> (w1326:dbl)
                        n380 = local read "rf step length 4"() -> (w1323:dbl)
                        n381 = local read "rf step length 5"() -> (w1318:dbl)
                        n382 = local read "rf step length 6"() -> (w1315:dbl)
                        n383 = local read "rf step length 1"() -> (w1335:dbl)
                        n384 = local read "rf step length 2"() -> (w1331:dbl)
                        n385 = local read "rf step watt 4"() -> (w1322:dbl)
                        n386 = local read "rf step watt 5"() -> (w1319:dbl)
                        n387 = local read "rf step watt 6"() -> (w1314:dbl)
                        n388 = local read "rf step watt 1"() -> (w1336:dbl)
                        n389 = local read "rf step watt 2"() -> (w1330:dbl)
                        n390 = local read "rf step watt 3"() -> (w1327:dbl)
                        n391 = Equal To 0?(x=w1314) -> (x = 0?=w1313:bool)
                        n392 = Equal To 0?(x=w1315) -> (x = 0?=w1312:bool)
                        n393 = Equal To 0?(x=w1319) -> (x = 0?=w1317:bool)
                        n394 = Equal To 0?(x=w1336) -> (x = 0?=w1334:bool)
                        n395 = Equal To 0?(x=w1318) -> (x = 0?=w1316:bool)
                        n396 = Equal To 0?(x=w1330) -> (x = 0?=w1329:bool)
                        n397 = Equal To 0?(x=w1322) -> (x = 0?=w1321:bool)
                        n398 = Equal To 0?(x=w1335) -> (x = 0?=w1333:bool)
                        n399 = Equal To 0?(x=w1327) -> (x = 0?=w1325:bool)
                        n400 = Equal To 0?(x=w1323) -> (x = 0?=w1320:bool)
                        n401 = Equal To 0?(x=w1331) -> (x = 0?=w1328:bool)
                        n402 = Equal To 0?(x=w1326) -> (x = 0?=w1324:bool)
                        n403 = Compound Arithmetic op=OR(w1334, w1333, w1329, w1328, w1325, w1324, w1321, w1320, w1317, w1316, w1313, w1312) -> (w1332:bool)
                      }
                      frame 7 {
                        n404 = local read "rf step length 5"() -> (w1347:dbl)
                        n405 = local read "rf step length 6"() -> (w1344:dbl)
                        n406 = local read "rf step length 7"() -> (w1339:dbl)
                        n407 = local read "rf step length 1"() -> (w1364:dbl)
                        n408 = local read "rf step length 2"() -> (w1360:dbl)
                        n409 = local read "rf step length 3"() -> (w1355:dbl)
                        n410 = local read "rf step length 4"() -> (w1352:dbl)
                        n411 = local read "rf step watt 5"() -> (w1348:dbl)
                        n412 = local read "rf step watt 6"() -> (w1343:dbl)
                        n413 = local read "rf step watt 7"() -> (w1340:dbl)
                        n414 = local read "rf step watt 1"() -> (w1365:dbl)
                        n415 = local read "rf step watt 2"() -> (w1359:dbl)
                        n416 = local read "rf step watt 3"() -> (w1356:dbl)
                        n417 = local read "rf step watt 4"() -> (w1351:dbl)
                        n418 = Equal To 0?(x=w1365) -> (x = 0?=w1363:bool)
                        n419 = Equal To 0?(x=w1364) -> (x = 0?=w1362:bool)
                        n420 = Equal To 0?(x=w1359) -> (x = 0?=w1358:bool)
                        n421 = Equal To 0?(x=w1360) -> (x = 0?=w1357:bool)
                        n422 = Equal To 0?(x=w1356) -> (x = 0?=w1354:bool)
                        n423 = Equal To 0?(x=w1355) -> (x = 0?=w1353:bool)
                        n424 = Equal To 0?(x=w1351) -> (x = 0?=w1350:bool)
                        n425 = Equal To 0?(x=w1352) -> (x = 0?=w1349:bool)
                        n426 = Equal To 0?(x=w1348) -> (x = 0?=w1346:bool)
                        n427 = Equal To 0?(x=w1347) -> (x = 0?=w1345:bool)
                        n428 = Equal To 0?(x=w1343) -> (x = 0?=w1342:bool)
                        n429 = Equal To 0?(x=w1344) -> (x = 0?=w1341:bool)
                        n430 = Equal To 0?(x=w1340) -> (x = 0?=w1338:bool)
                        n431 = Equal To 0?(x=w1339) -> (x = 0?=w1337:bool)
                        n432 = Compound Arithmetic op=OR(w1363, w1362, w1358, w1357, w1354, w1353, w1350, w1349, w1346, w1345, w1342, w1341, w1338, w1337) -> (w1361:bool)
                      }
                      frame 8 {
                        n433 = local read "rf step length 6"() -> (w1377:dbl)
                        n434 = local read "rf step length 7"() -> (w1372:dbl)
                        n435 = local read "rf step length 8"() -> (w1369:dbl)
                        n436 = local read "rf step length 5"() -> (w1380:dbl)
                        n437 = local read "rf step length 1"() -> (w1397:dbl)
                        n438 = local read "rf step length 4"() -> (w1385:dbl)
                        n439 = local read "rf step length 2"() -> (w1393:dbl)
                        n440 = local read "rf step length 3"() -> (w1388:dbl)
                        n441 = local read "rf step watt 6"() -> (w1376:dbl)
                        n442 = local read "rf step watt 7"() -> (w1373:dbl)
                        n443 = local read "rf step watt 8"() -> (w1368:dbl)
                        n444 = local read "rf step watt 5"() -> (w1381:dbl)
                        n445 = local read "rf step watt 1"() -> (w1398:dbl)
                        n446 = local read "rf step watt 2"() -> (w1392:dbl)
                        n447 = local read "rf step watt 4"() -> (w1384:dbl)
                        n448 = local read "rf step watt 3"() -> (w1389:dbl)
                        n449 = Equal To 0?(x=w1376) -> (x = 0?=w1375:bool)
                        n450 = Equal To 0?(x=w1373) -> (x = 0?=w1371:bool)
                        n451 = Equal To 0?(x=w1377) -> (x = 0?=w1374:bool)
                        n452 = Equal To 0?(x=w1372) -> (x = 0?=w1370:bool)
                        n453 = Equal To 0?(x=w1368) -> (x = 0?=w1367:bool)
                        n454 = Equal To 0?(x=w1381) -> (x = 0?=w1379:bool)
                        n455 = Equal To 0?(x=w1369) -> (x = 0?=w1366:bool)
                        n456 = Equal To 0?(x=w1398) -> (x = 0?=w1396:bool)
                        n457 = Equal To 0?(x=w1380) -> (x = 0?=w1378:bool)
                        n458 = Equal To 0?(x=w1392) -> (x = 0?=w1391:bool)
                        n459 = Equal To 0?(x=w1384) -> (x = 0?=w1383:bool)
                        n460 = Equal To 0?(x=w1397) -> (x = 0?=w1395:bool)
                        n461 = Equal To 0?(x=w1389) -> (x = 0?=w1387:bool)
                        n462 = Equal To 0?(x=w1385) -> (x = 0?=w1382:bool)
                        n463 = Equal To 0?(x=w1393) -> (x = 0?=w1390:bool)
                        n464 = Equal To 0?(x=w1388) -> (x = 0?=w1386:bool)
                        n465 = Compound Arithmetic op=OR(w1396, w1395, w1391, w1390, w1387, w1386, w1383, w1382, w1379, w1378, w1375, w1374, w1371, w1370, w1367, w1366) -> (w1394:bool)
                      }
                      frame 9 {
                        n466 = local read "rf step length 1"() -> (w1434:dbl)
                        n467 = local read "rf step length 2"() -> (w1430:dbl)
                        n468 = local read "rf step length 3"() -> (w1425:dbl)
                        n469 = local read "rf step length 4"() -> (w1422:dbl)
                        n470 = local read "rf step length 5"() -> (w1417:dbl)
                        n471 = local read "rf step length 6"() -> (w1414:dbl)
                        n472 = local read "rf step length 7"() -> (w1409:dbl)
                        n473 = local read "rf step length 8"() -> (w1406:dbl)
                        n474 = local read "rf step length 9"() -> (w1401:dbl)
                        n475 = local read "rf step watt 1"() -> (w1435:dbl)
                        n476 = local read "rf step watt 2"() -> (w1429:dbl)
                        n477 = local read "rf step watt 3"() -> (w1426:dbl)
                        n478 = local read "rf step watt 4"() -> (w1421:dbl)
                        n479 = local read "rf step watt 5"() -> (w1418:dbl)
                        n480 = local read "rf step watt 6"() -> (w1413:dbl)
                        n481 = local read "rf step watt 7"() -> (w1410:dbl)
                        n482 = local read "rf step watt 8"() -> (w1405:dbl)
                        n483 = local read "rf step watt 9"() -> (w1402:dbl)
                        n484 = Equal To 0?(x=w1435) -> (x = 0?=w1433:bool)
                        n485 = Equal To 0?(x=w1434) -> (x = 0?=w1432:bool)
                        n486 = Equal To 0?(x=w1429) -> (x = 0?=w1428:bool)
                        n487 = Equal To 0?(x=w1430) -> (x = 0?=w1427:bool)
                        n488 = Equal To 0?(x=w1426) -> (x = 0?=w1424:bool)
                        n489 = Equal To 0?(x=w1425) -> (x = 0?=w1423:bool)
                        n490 = Equal To 0?(x=w1421) -> (x = 0?=w1420:bool)
                        n491 = Equal To 0?(x=w1422) -> (x = 0?=w1419:bool)
                        n492 = Equal To 0?(x=w1418) -> (x = 0?=w1416:bool)
                        n493 = Equal To 0?(x=w1417) -> (x = 0?=w1415:bool)
                        n494 = Equal To 0?(x=w1413) -> (x = 0?=w1412:bool)
                        n495 = Equal To 0?(x=w1414) -> (x = 0?=w1411:bool)
                        n496 = Equal To 0?(x=w1410) -> (x = 0?=w1408:bool)
                        n497 = Equal To 0?(x=w1409) -> (x = 0?=w1407:bool)
                        n498 = Equal To 0?(x=w1405) -> (x = 0?=w1404:bool)
                        n499 = Equal To 0?(x=w1406) -> (x = 0?=w1403:bool)
                        n500 = Equal To 0?(x=w1402) -> (x = 0?=w1400:bool)
                        n501 = Equal To 0?(x=w1401) -> (x = 0?=w1399:bool)
                        n502 = Compound Arithmetic op=OR(w1433, w1432, w1428, w1427, w1424, w1423, w1420, w1419, w1416, w1415, w1412, w1411, w1408, w1407, w1404, w1403, w1400, w1399) -> (w1431:bool)
                      }
                      frame 10 {
                        n503 = local read "rf step length 10"() -> (w1439:dbl)
                        n504 = local read "rf step length 1"() -> (w1475:dbl)
                        n505 = local read "rf step length 2"() -> (w1471:dbl)
                        n506 = local read "rf step length 3"() -> (w1466:dbl)
                        n507 = local read "rf step length 4"() -> (w1463:dbl)
                        n508 = local read "rf step length 5"() -> (w1458:dbl)
                        n509 = local read "rf step length 6"() -> (w1455:dbl)
                        n510 = local read "rf step length 7"() -> (w1450:dbl)
                        n511 = local read "rf step length 8"() -> (w1447:dbl)
                        n512 = local read "rf step length 9"() -> (w1442:dbl)
                        n513 = local read "rf step watt 10"() -> (w1438:dbl)
                        n514 = local read "rf step watt 1"() -> (w1476:dbl)
                        n515 = local read "rf step watt 2"() -> (w1470:dbl)
                        n516 = local read "rf step watt 3"() -> (w1467:dbl)
                        n517 = local read "rf step watt 4"() -> (w1462:dbl)
                        n518 = local read "rf step watt 5"() -> (w1459:dbl)
                        n519 = local read "rf step watt 6"() -> (w1454:dbl)
                        n520 = local read "rf step watt 7"() -> (w1451:dbl)
                        n521 = local read "rf step watt 8"() -> (w1446:dbl)
                        n522 = local read "rf step watt 9"() -> (w1443:dbl)
                        n523 = Equal To 0?(x=w1438) -> (x = 0?=w1437:bool)
                        n524 = Equal To 0?(x=w1439) -> (x = 0?=w1436:bool)
                        n525 = Equal To 0?(x=w1476) -> (x = 0?=w1474:bool)
                        n526 = Equal To 0?(x=w1475) -> (x = 0?=w1473:bool)
                        n527 = Equal To 0?(x=w1470) -> (x = 0?=w1469:bool)
                        n528 = Equal To 0?(x=w1471) -> (x = 0?=w1468:bool)
                        n529 = Equal To 0?(x=w1467) -> (x = 0?=w1465:bool)
                        n530 = Equal To 0?(x=w1466) -> (x = 0?=w1464:bool)
                        n531 = Equal To 0?(x=w1462) -> (x = 0?=w1461:bool)
                        n532 = Equal To 0?(x=w1463) -> (x = 0?=w1460:bool)
                        n533 = Equal To 0?(x=w1459) -> (x = 0?=w1457:bool)
                        n534 = Equal To 0?(x=w1458) -> (x = 0?=w1456:bool)
                        n535 = Equal To 0?(x=w1454) -> (x = 0?=w1453:bool)
                        n536 = Equal To 0?(x=w1455) -> (x = 0?=w1452:bool)
                        n537 = Equal To 0?(x=w1451) -> (x = 0?=w1449:bool)
                        n538 = Equal To 0?(x=w1450) -> (x = 0?=w1448:bool)
                        n539 = Equal To 0?(x=w1446) -> (x = 0?=w1445:bool)
                        n540 = Equal To 0?(x=w1447) -> (x = 0?=w1444:bool)
                        n541 = Equal To 0?(x=w1443) -> (x = 0?=w1441:bool)
                        n542 = Equal To 0?(x=w1442) -> (x = 0?=w1440:bool)
                        n543 = Compound Arithmetic op=OR(w1474, w1473, w1469, w1468, w1465, w1464, w1461, w1460, w1457, w1456, w1453, w1452, w1449, w1448, w1445, w1444, w1441, w1440, w1437, w1436) -> (w1472:bool)
                      }
                    }
                  }
                }
              }
              frame 1 {
                # "multilayer recipe"
              }
            }
            n544 = local read "power rf"() -> (w969:dbl)
            n545 = Equal To 0?(x=w969) -> ()  [unwired: 1 out]
            n546 = local read "Pressure set mbar"() -> (w972:dbl)
            n547 = local read "total length error"() -> (w974:bool)
            n548 = local read "Ar set sccm"() -> (w973:dbl)
            n549 = Equal To 0?(x=w973) -> (x = 0?=w971:bool)
            n550 = Equal To 0?(x=w972) -> (x = 0?=w970:bool)
            n551 = Build Array(FALSE, w990, w989, w987, w986, w985, w984, w983, w978, w977, w976, w974, w971, w970) -> (w975:bool[])
            n552 = Boolean Array To Number(Boolean array=w975) -> (number=w993:u32)
            n553 = Mantissa & Exponent(0:w993) -> (2:w992:dbl)  [unwired: 1 out]
            n554 = case shown="11" w992 {
              tunnel: [TRUE FALSE FALSE FALSE FALSE FALSE FALSE FALSE FALSE FALSE FALSE FALSE FALSE FALSE] -> w982
              frame 0, Default {
              }
              frame 1 {
                n555 = One Button Dialog(message="Enter Recipe Name !") -> ()  [unwired: 1 in, 1 out]
              }
              frame 2 {
                n556 = One Button Dialog(message="Enter Substrate Material !") -> ()  [unwired: 1 in, 1 out]
              }
              frame 3 {
                n557 = One Button Dialog(message="Enter Core Diameter !") -> ()  [unwired: 1 in, 1 out]
              }
              frame 4 {
                n558 = One Button Dialog(message="Enter Left Initial Diameter !") -> ()  [unwired: 1 in, 1 out]
              }
              frame 5 {
                n559 = One Button Dialog(message="Enter Web Thickness !") -> ()  [unwired: 1 in, 1 out]
              }
              frame 6 {
                n560 = One Button Dialog(message="Enter Web Speed !") -> ()  [unwired: 1 in, 1 out]
              }
              frame 7 {
                n561 = One Button Dialog(message="Enter Tension Value !") -> ()  [unwired: 1 in, 1 out]
              }
              frame 8 {
                n562 = One Button Dialog(message="Enter Microwave Power !") -> ()  [unwired: 1 in, 1 out]
              }
              frame 9 {
                n563 = One Button Dialog(message="Check DC Step Length(s) and Power(s) !") -> ()  [unwired: 1 in, 1 out]
              }
              frame 10 {
                n564 = One Button Dialog(message="Enter RF Power !") -> ()  [unwired: 1 in, 1 out]
              }
              frame 11 {
                n565 = One Button Dialog(message="Check Step Length(s) !") -> ()  [unwired: 1 in, 1 out]
              }
              frame 12 {
                n566 = One Button Dialog(message="Enter Argon Flow !") -> ()  [unwired: 1 in, 1 out]
              }
              frame 13 {
                n567 = One Button Dialog(message="Enter Pressure  !") -> ()  [unwired: 1 in, 1 out]
              }
            }
            "done" <- w982
          }
        }
        n568 = case shown="True" "CALCULATE" {
          frame False {
          }
          frame True {
            n569 = stacked-sequence {
              frame #0 {
                n570 = local write "total length"(0.0 ("total length")) -> ()
                "left diameter after roll" <- "left initial diameter"
              }
              frame #1 {
                n571 = while {
                  i -> [w958]
                  stop <- w957 stop-if-true
                  n572 = local read "left diameter after roll"() -> (w956:dbl)
                  n573 = local read "web thickness"() -> (w954:dbl)
                  n574 = Wait Until Next ms Multiple(millisecond multiple=u32 100) -> ()  [unwired: 1 out]
                  n575 = local read "core diameter"() -> (w953:dbl)
                  n576 = Multiply(x=w954, y=0.002) -> (x*y=w964:dbl)
                  n577 = Multiply(x=3.141592653589793, y=w956) -> (x*y=w947:dbl)
                  n578 = Subtract(x=w956, y=w964) -> (x-y=w963:dbl)
                  n579 = local read "CALCULATE"() -> (w950:bool)
                  n580 = local write "left diameter after roll"(w963) -> ()
                  n581 = Divide(x=w947, y=10.0) -> (x/y=w949:dbl)
                  n582 = Less Or Equal?(x=w963, y=w953) -> (x <= y?=w959:bool)
                  n583 = local read "total length"() -> (w961:dbl)
                  n584 = Not(x=w950) -> (.not. x?=w951:bool)
                  n585 = Greater Or Equal?(x=w958, y=600) -> (x >= y?=w955:bool)
                  n586 = Add(x=w949, y=w961) -> (x+y=w962:dbl)
                  n587 = local write "total length"(w962) -> ()
                  n588 = Compound Arithmetic op=OR(w959, w955, w951) -> (w957:bool)
                }
              }
              frame #2 {
                n589 = local write "CALCULATE"(FALSE ("CALCULATE")) -> ()
              }
            }
          }
        }
        n590 = local read "single process selection"() -> (w894:enum32{"microwave", "dcsputter", "rfsputter"})
        n591 = local read "Recipe Selection"() -> (w906:u16)
        n592 = local read "Web Selection"() -> (w902:u16)
        n593 = Equal?(x=w906, y=u16 1) -> (x = y?=w904:bool)
        n594 = Equal?(x=w902, y=u16 1) -> (x = y?=w901:bool)
        n595 = case shown="\"rfsputter\"" w894 {
          tunnel: [T3."Microwave                " ("single process selection") T3."DC Sputter                   " ("single process selection") T3."RF Sputter                         " ("single process selection")] -> w893
          tunnel: [FALSE TRUE FALSE] -> w891
          tunnel: [FALSE FALSE TRUE] -> w890
          frame "microwave", Default {
          }
          frame "dcsputter" {
          }
          frame "rfsputter" {
          }
        }
        n596 = case shown="True" w904 {
          tunnel: [T2."Single Recipe                                    " ("recipe selection") T2."Multilayer Recipe                                      " ("recipe selection")] -> w900
          frame False {
          }
          frame True {
          }
        }
        n597 = case shown="False" w901 {
          tunnel: [T1."Web                                                    " ("web-other tab") T1."Other                                                      " ("web-other tab")] -> w899
          frame False {
          }
          frame True {
          }
        }
        n598 = property on="recipe selection" class="TabCtl (strict)"("Value"=w900) -> ()  [unwired: 2 in, 2 out]
        n599 = property on="web-other tab" class="TabCtl (strict)"("Value"=w899) -> ()  [unwired: 2 in, 2 out]
        n600 = property on="single process selection" class="TabCtl (strict)"("Value"=w893) -> ()  [unwired: 2 in, 2 out]
        n601 = property on="steplist tab DC" class="TabCtl (strict)"("Visible"=w891) -> ()  [unwired: 2 in, 2 out]
        n602 = property on="steplist tab RF" class="TabCtl (strict)"("Visible"=w890) -> ()  [unwired: 2 in, 2 out]
        n603 = local read "single process selection"() -> (w889:enum32{"microwave", "dcsputter", "rfsputter"})
        n604 = case shown="\"dcsputter\"" w889 {
          tunnel: [0.0 w914 w928] -> w898
          frame "microwave", Default {
          }
          frame "rfsputter" {
            n605 = Compound Arithmetic op=ADD("rf step length 1", "rf step length 2", "rf step length 3", "rf step length 4", "rf step length 5", "rf step length 6", "rf step length 7", "rf step length 8", "rf step length 9", "rf step length 10") -> (w914:dbl)
          }
          frame "dcsputter" {
            n606 = Compound Arithmetic op=ADD("dc step length 1", "dc step length 2", "dc step length 3", "dc step length 4", "dc step length 5", "dc step length 6", "dc step length 7", "dc step length 8", "dc step length 9", "dc step length 10") -> (w928:dbl)
          }
        }
        n607 = case shown="True" "CANCEL" {
          tunnel: [FALSE w909] -> w886
          frame False {
          }
          frame True {
            n608 = stacked-sequence {
              tunnel: [_ TRUE] -> w909
              frame #0 {
                n609 = Wait (ms)(milliseconds to wait=u32 500) -> ()  [unwired: 1 out]
              }
              frame #1 {
                w912 = FALSE ("CALCULATE")
                n610 = local write "CANCEL"(w912) -> ()
                n611 = local write "CALCULATE"(w912) -> ()
              }
            }
          }
        }
        n612 = local read "total length"() -> (w895:dbl)
        n613 = local read "done"() -> (w888:bool)
        n614 = Greater?(x=w898, y=w895) -> ()  [unwired: 1 out]
        n615 = Compound Arithmetic op=OR(w888, w886) -> (w896:bool)
        "total length error" <- FALSE ("total length error")
      }
      n616 = while {
        stop <- w343 stop-if-true
        n617 = local read "done"() -> (w340:bool)
        n618 = Wait Until Next ms Multiple(millisecond multiple=u32 300) -> ()  [unwired: 1 out]
        n619 = case shown="True" w340 {
          tunnel: [FALSE w348] -> w342
          frame False {
          }
          frame True {
            n620 = stacked-sequence {
              seq-local: [w377 _ _ _ _ _ _ _] -> [_ w453 _ _ _ _ _ _]
              seq-local: [_ w451 _ _ _ _ _ _] -> [_ _ w564 _ _ _ _ _]
              seq-local: [_ _ w563 _ _ _ _ _] -> [_ _ _ w592 _ _ _ _]
              seq-local: [_ _ _ w591 _ _ _ _] -> [_ _ _ _ w665 _ _ _]
              seq-local: [_ _ _ _ w664 _ _ _] -> [_ _ _ _ _ w803 _ _]
              seq-local: [_ _ _ _ _ w802 _ _] -> [_ _ _ _ _ _ w868 _]
              tunnel: [_ _ _ _ _ _ _ TRUE] -> w348
              frame #0 {
                w355 = "\t"
                w362 = "\t"
                w369 = "\t"
                w373 = "\t"
                w380 = "\r\n"
                w388 = "\r\n"
                w389 = "\t"
                n621 = local read "Recipe Selection"() -> (w386:u16)
                n622 = local read "Web Selection"() -> (w383:u16)
                n623 = Equal?(x=w386, y=u16 0) -> (x = y?=w385:bool)
                n624 = Equal?(x=w383, y=u16 0) -> (x = y?=w384:bool)
                n625 = local read "core diameter"() -> (w378:dbl)
                n626 = case shown="False" w385 {
                  tunnel: ["Multilayer Recipe" ("string") "Single Recipe" ("string")] -> w359
                  frame False {
                  }
                  frame True {
                  }
                }
                n627 = case shown="False" w384 {
                  tunnel: ["Other" ("string") "Web" ("string")] -> w353
                  frame False {
                  }
                  frame True {
                  }
                }
                n628 = local read "Substrate Material"() -> (w370:string)
                n629 = Number To Decimal String(number=w378) -> (decimal integer string=w349:string)  [unwired: 1 in]
                n630 = local read "Recipe Name"() -> (w391:string)
                n631 = Concatenate Strings(w380, w380) -> (w379:string)
                n632 = Concatenate Strings("Core Diameter(mm)" ("string"), w369, w369, w369, ":" ("string"), "\t", w349, "\r\n") -> (w351:string)
                n633 = Concatenate Strings(w388, w388) -> (w381:string)
                n634 = Concatenate Strings("Recipe Selection" ("string"), w362, w362, w362, ":" ("string"), "\t", w359, "\r\n") -> (w361:string)
                n635 = Concatenate Strings("Recipe Name" ("string"), w389, w389, w389, ":" ("string"), "\t", w391, "\r\n") -> (w392:string)
                n636 = Concatenate Strings("Substrate Material" ("string"), w373, w373, w373, ":" ("string"), "\t", w370, "\r\n") -> (w371:string)
                n637 = Concatenate Strings("Web Selection" ("string"), w355, w355, w355, ":" ("string"), "\t", w353, "\r\n") -> (w352:string)
                n638 = Concatenate Strings(w392, w371, w381, w361, w352, w379, w351) -> (w377:string)
              }
              frame #1 {
                w409 = "\t"
                w416 = "\t"
                w423 = "\t"
                w430 = "\t"
                w437 = "\t"
                w443 = "\t"
                w445 = "\r\n"
                w455 = "\r\n"
                w457 = "\r\n"
                n639 = local read "single process selection"() -> (w447:enum32{"microwave", "dcsputter", "rfsputter"})
                n640 = local read "web thickness"() -> (w450:dbl)
                n641 = local read "left initial diameter"() -> (w401:dbl)
                n642 = case shown="\"dcsputter\"" w447 {
                  tunnel: ["Microwave" ("string") "DC Sputter" ("string") "RF Sputter" ("string")] -> w410
                  tunnel: [FALSE TRUE FALSE] -> w446
                  frame "microwave", Default {
                  }
                  frame "dcsputter" {
                  }
                  frame "rfsputter" {
                  }
                }
                n643 = local read "web speed"() -> (w449:dbl)
                n644 = local read "tension value"() -> (w448:dbl)
                n645 = Number To Decimal String(number=w450) -> (decimal integer string=w433:string)  [unwired: 1 in]
                n646 = Format Into String(format string="%.;%f", w401) -> (resulting string=w400:string)  [unwired: 2 in, 1 out]
                n647 = Number To Decimal String(number=w449) -> (decimal integer string=w424:string)  [unwired: 1 in]
                n648 = Number To Decimal String(number=w448) -> (decimal integer string=w417:string)  [unwired: 1 in]
                n649 = Concatenate Strings(w455, w455) -> (w454:string)
                n650 = Concatenate Strings("Web Thickness(µm)" ("string"), w437, w437, w437, ":" ("string"), "\t", w433, "\r\n") -> (w432:string)
                n651 = case shown="True" w446 {
                  tunnel: ["NULL" ("string") w459] -> w403
                  frame False {
                  }
                  frame True {
                    n652 = local read "DC Sputter Chamber Selection"() -> (w460:enum32{"chamber II", "chamber III"})
                    n653 = case shown="\"chamber II\", Default" w460 {
                      tunnel: ["II" ("string") "III" ("string")] -> w459
                      frame "chamber II", Default {
                      }
                      frame "chamber III" {
                      }
                    }
                  }
                }
                n654 = Concatenate Strings(w457, w457) -> (w456:string)
                n655 = Concatenate Strings("Web Speed(cm/min)" ("string"), w430, w430, w430, ":" ("string"), "\t", w424, "\r\n") -> (w426:string)
                n656 = Concatenate Strings("Tension Value(N)" ("string"), w423, w423, w423, ":" ("string"), "\t", w417, "\r\n") -> (w419:string)
                n657 = Concatenate Strings("Left Initial Diameter(mm)" ("string"), w443, w443, w443, ":" ("string"), "\t", w400, "\r\n") -> (w439:string)
                n658 = Concatenate Strings("Single Process Selection" ("string"), w416, w416, w416, ":" ("string"), "\t", w410, "\r\n") -> (w412:string)
                n659 = Concatenate Strings(w445, w445) -> (w444:string)
                n660 = Concatenate Strings("Chamber Selection" ("string"), w409, w409, w409, ":" ("string"), "\t", w403, "\r\n") -> (w405:string)
                n661 = Concatenate Strings(w439, w432, w456, w426, w419, w454, w412, w405, w444) -> (w452:string)
                n662 = Concatenate Strings(w453, w452) -> (w451:string)
              }
              frame #2 {
                w477 = "\t"
                w469 = "\t"
                w522 = "\t"
                w536 = "\t"
                w541 = "\t"
                w533 = "\t"
                w528 = "\t"
                w549 = "\t"
                w544 = "\t"
                w552 = "\t"
                w557 = "\t"
                w560 = "\r\n"
                w562 = "\r\n"
                w568 = "\r\n"
                n663 = local read "dc step watt 4"() -> (w547:dbl)
                n664 = local read "dc step watt 1"() -> (w555:dbl)
                n665 = local read "dc step watt 2"() -> (w554:dbl)
                n666 = local read "dc step watt 3"() -> (w546:dbl)
                n667 = local read "dc step watt 5"() -> (w524:dbl)
                n668 = Number To Decimal String(number=w547) -> (decimal integer string=w491:string)  [unwired: 1 in]
                n669 = Number To Decimal String(number=w554) -> (decimal integer string=w495:string)  [unwired: 1 in]
                n670 = Number To Decimal String(number=w546) -> (decimal integer string=w493:string)  [unwired: 1 in]
                n671 = Number To Decimal String(number=w555) -> (decimal integer string=w497:string)  [unwired: 1 in]
                n672 = Number To Decimal String(number=w524) -> (decimal integer string=w489:string)  [unwired: 1 in]
                n673 = local read "power microwave"() -> (w566:dbl)
                n674 = Number To Decimal String(number=w566) -> (decimal integer string=w472:string)  [unwired: 1 in]
                n675 = Concatenate Strings("DC Step 4 power" ("string"), w549, w549, w549, ":" ("string"), "\t", w491, "\r\n") -> (w517:string)
                n676 = Concatenate Strings("DC Step 5 power" ("string"), w522, w522, w522, ":" ("string"), "\t", w489, "\r\n") -> (w516:string)
                n677 = Concatenate Strings("DC Step 2 power" ("string"), w552, w552, w552, ":" ("string"), "\t", w495, "\r\n") -> (w519:string)
                n678 = Concatenate Strings("DC Step 3 power" ("string"), w544, w544, w544, ":" ("string"), "\t", w493, "\r\n") -> (w518:string)
                n679 = Concatenate Strings("DC Step 1 power" ("string"), w557, w557, w557, ":" ("string"), "\t", w497, "\r\n") -> (w520:string)
                n680 = Concatenate Strings("DC Power Steps(power-length)" ("string"), w560, w560) -> (w559:string)
                n681 = Concatenate Strings(w520, w519, w518, w517, w516) -> (w509:string)
                n682 = Concatenate Strings(w568, w568) -> (w567:string)
                n683 = Concatenate Strings(w562, w562) -> (w478:string)
                n684 = Concatenate Strings("Microwave Power(watt)" ("string"), w477, w477, w477, ":" ("string"), "\t", w472, "\r\n") -> (w473:string)
                n685 = local read "dc step watt 10"() -> (w525:dbl)
                n686 = local read "dc step watt 9"() -> (w538:dbl)
                n687 = local read "dc step watt 7"() -> (w531:dbl)
                n688 = local read "dc step watt 8"() -> (w539:dbl)
                n689 = local read "dc step watt 6"() -> (w530:dbl)
                n690 = Number To Decimal String(number=w538) -> (decimal integer string=w485:string)  [unwired: 1 in]
                n691 = Number To Decimal String(number=w525) -> (decimal integer string=w487:string)  [unwired: 1 in]
                n692 = Number To Decimal String(number=w531) -> (decimal integer string=w481:string)  [unwired: 1 in]
                n693 = Number To Decimal String(number=w539) -> (decimal integer string=w483:string)  [unwired: 1 in]
                n694 = Number To Decimal String(number=w530) -> (decimal integer string=w479:string)  [unwired: 1 in]
                n695 = Concatenate Strings("DC Step 9 power" ("string"), w536, w536, w536, ":" ("string"), "\t", w485, "\r\n") -> (w512:string)
                n696 = Concatenate Strings("DC Step 10 power" ("string"), w469, w469, w469, ":" ("string"), "\t", w487, "\r\n") -> (w511:string)
                n697 = Concatenate Strings("DC Step 7 power" ("string"), w533, w533, w533, ":" ("string"), "\t", w481, "\r\n") -> (w514:string)
                n698 = Concatenate Strings("DC Step 8 power" ("string"), w541, w541, w541, ":" ("string"), "\t", w483, "\r\n") -> (w513:string)
                n699 = Concatenate Strings("DC Step 6 power" ("string"), w528, w528, w528, ":" ("string"), "\t", w479, "\r\n") -> (w515:string)
                n700 = Concatenate Strings(w515, w514, w513, w512, w511) -> (w510:string)
                n701 = Concatenate Strings(w473, w478, w567, w559, w509, w510) -> (w565:string)
                n702 = Concatenate Strings(w564, w565) -> (w563:string)
              }
              frame #3 {
                w589 = "\r\n"
                w569 = "\t"
                w580 = "\t"
                w572 = "\t"
                w574 = "\t"
                w576 = "\t"
                w577 = "\t"
                w582 = "\t"
                w584 = "\t"
                w587 = "\t"
                w586 = "\t"
                n703 = local read "dc step length 10"() -> (w636:dbl)
                n704 = local read "dc step length 9"() -> (w643:dbl)
                n705 = local read "dc step length 7"() -> (w640:dbl)
                n706 = local read "dc step length 8"() -> (w644:dbl)
                n707 = local read "dc step length 6"() -> (w639:dbl)
                n708 = local read "dc step length 4"() -> (w648:dbl)
                n709 = local read "dc step length 2"() -> (w651:dbl)
                n710 = local read "dc step length 3"() -> (w647:dbl)
                n711 = local read "dc step length 1"() -> (w652:dbl)
                n712 = local read "dc step length 5"() -> (w635:dbl)
                n713 = Number To Decimal String(number=w643) -> (decimal integer string=w599:string)  [unwired: 1 in]
                n714 = Number To Decimal String(number=w636) -> (decimal integer string=w601:string)  [unwired: 1 in]
                n715 = Number To Decimal String(number=w640) -> (decimal integer string=w595:string)  [unwired: 1 in]
                n716 = Number To Decimal String(number=w644) -> (decimal integer string=w597:string)  [unwired: 1 in]
                n717 = Number To Decimal String(number=w639) -> (decimal integer string=w593:string)  [unwired: 1 in]
                n718 = Number To Decimal String(number=w648) -> (decimal integer string=w605:string)  [unwired: 1 in]
                n719 = Number To Decimal String(number=w651) -> (decimal integer string=w609:string)  [unwired: 1 in]
                n720 = Number To Decimal String(number=w647) -> (decimal integer string=w607:string)  [unwired: 1 in]
                n721 = Number To Decimal String(number=w652) -> (decimal integer string=w611:string)  [unwired: 1 in]
                n722 = Number To Decimal String(number=w635) -> (decimal integer string=w603:string)  [unwired: 1 in]
                n723 = Concatenate Strings("DC Step 9 length" ("string"), w572, w572, w572, ":" ("string"), "\t", w599, "\r\n") -> (w625:string)
                n724 = Concatenate Strings("DC Step 10 length" ("string"), w569, w569, w569, ":" ("string"), "\t", w601, "\r\n") -> (w624:string)
                n725 = Concatenate Strings("DC Step 7 length" ("string"), w576, w576, w576, ":" ("string"), "\t", w595, "\r\n") -> (w627:string)
                n726 = Concatenate Strings("DC Step 8 length" ("string"), w574, w574, w574, ":" ("string"), "\t", w597, "\r\n") -> (w626:string)
                n727 = Concatenate Strings("DC Step 6 length" ("string"), w577, w577, w577, ":" ("string"), "\t", w593, "\r\n") -> (w628:string)
                n728 = Concatenate Strings("DC Step 4 length" ("string"), w582, w582, w582, ":" ("string"), "\t", w605, "\r\n") -> (w630:string)
                n729 = Concatenate Strings("DC Step 5 length" ("string"), w580, w580, w580, ":" ("string"), "\t", w603, "\r\n") -> (w629:string)
                n730 = Concatenate Strings("DC Step 2 length" ("string"), w587, w587, w587, ":" ("string"), "\t", w609, "\r\n") -> (w632:string)
                n731 = Concatenate Strings("DC Step 3 length" ("string"), w584, w584, w584, ":" ("string"), "\t", w607, "\r\n") -> (w631:string)
                n732 = Concatenate Strings("DC Step 1 length" ("string"), w586, w586, w586, ":" ("string"), "\t", w611, "\r\n") -> (w633:string)
                n733 = Concatenate Strings(w628, w627, w626, w625, w624) -> (w623:string)
                n734 = Concatenate Strings(w633, w632, w631, w630, w629) -> (w590:string)
                n735 = Concatenate Strings(w589, w589, w590, w623) -> (w654:string)
                n736 = Concatenate Strings(w592, w654) -> (w591:string)
              }
              frame #4 {
                w660 = "\r\n"
                w662 = "\r\n"
                w656 = "\t"
                w709 = "\t"
                w704 = "\t"
                w699 = "\t"
                w694 = "\t"
                w689 = "\t"
                w684 = "\t"
                w679 = "\t"
                w674 = "\t"
                w669 = "\t"
                n737 = local read "rf step watt 10"() -> (w735:dbl)
                n738 = local read "rf step watt 9"() -> (w738:dbl)
                n739 = local read "rf step watt 7"() -> (w737:dbl)
                n740 = local read "rf step watt 8"() -> (w739:dbl)
                n741 = local read "rf step watt 6"() -> (w736:dbl)
                n742 = local read "rf step watt 4"() -> (w741:dbl)
                n743 = local read "rf step watt 2"() -> (w742:dbl)
                n744 = local read "rf step watt 3"() -> (w740:dbl)
                n745 = local read "rf step watt 1"() -> (w743:dbl)
                n746 = local read "rf step watt 5"() -> (w734:dbl)
                n747 = Number To Decimal String(number=w738) -> (decimal integer string=w717:string)  [unwired: 1 in]
                n748 = Number To Decimal String(number=w735) -> (decimal integer string=w718:string)  [unwired: 1 in]
                n749 = Number To Decimal String(number=w737) -> (decimal integer string=w715:string)  [unwired: 1 in]
                n750 = Number To Decimal String(number=w739) -> (decimal integer string=w716:string)  [unwired: 1 in]
                n751 = Number To Decimal String(number=w736) -> (decimal integer string=w714:string)  [unwired: 1 in]
                n752 = Number To Decimal String(number=w741) -> (decimal integer string=w720:string)  [unwired: 1 in]
                n753 = Number To Decimal String(number=w742) -> (decimal integer string=w722:string)  [unwired: 1 in]
                n754 = Number To Decimal String(number=w740) -> (decimal integer string=w721:string)  [unwired: 1 in]
                n755 = Number To Decimal String(number=w743) -> (decimal integer string=w723:string)  [unwired: 1 in]
                n756 = Number To Decimal String(number=w734) -> (decimal integer string=w719:string)  [unwired: 1 in]
                n757 = Concatenate Strings("RF Step 9 power" ("string"), w704, w704, w704, ":" ("string"), "\t", w717, "\r\n") -> (w725:string)
                n758 = Concatenate Strings("RF Step 10 power" ("string"), w656, w656, w656, ":" ("string"), "\t", w718, "\r\n") -> (w724:string)
                n759 = Concatenate Strings("RF Step 7 power" ("string"), w694, w694, w694, ":" ("string"), "\t", w715, "\r\n") -> (w727:string)
                n760 = Concatenate Strings("RF Step 8 power" ("string"), w699, w699, w699, ":" ("string"), "\t", w716, "\r\n") -> (w726:string)
                n761 = Concatenate Strings("RF Step 6 power" ("string"), w689, w689, w689, ":" ("string"), "\t", w714, "\r\n") -> (w728:string)
                n762 = Concatenate Strings("RF Step 4 power" ("string"), w684, w684, w684, ":" ("string"), "\t", w720, "\r\n") -> (w730:string)
                n763 = Concatenate Strings("RF Step 5 power" ("string"), w709, w709, w709, ":" ("string"), "\t", w719, "\r\n") -> (w729:string)
                n764 = Concatenate Strings("RF Step 2 power" ("string"), w674, w674, w674, ":" ("string"), "\t", w722, "\r\n") -> (w732:string)
                n765 = Concatenate Strings("RF Step 3 power" ("string"), w679, w679, w679, ":" ("string"), "\t", w721, "\r\n") -> (w731:string)
                n766 = Concatenate Strings("RF Step 1 power" ("string"), w669, w669, w669, ":" ("string"), "\t", w723, "\r\n") -> (w733:string)
                n767 = Concatenate Strings("RF Power Steps(power-length)" ("string"), w660, w660) -> (w659:string)
                n768 = Concatenate Strings(w733, w732, w731, w730, w729) -> (w658:string)
                n769 = Concatenate Strings(w728, w727, w726, w725, w724) -> (w657:string)
                n770 = Concatenate Strings(w662, w662, w659, w658, w657) -> (w663:string)
                n771 = Concatenate Strings(w665, w663) -> (w664:string)
              }
              frame #5 {
                w749 = "\t"
                w756 = "\r\n"
                w760 = "\t"
                w767 = "\r\n"
                w770 = "\t"
                w779 = "\t"
                w804 = "\r\n"
                w800 = "\t"
                w790 = "\t"
                w797 = "\t"
                w795 = "\t"
                w794 = "\t"
                w792 = "\t"
                w787 = "\t"
                w785 = "\t"
                w783 = "\t"
                w782 = "\t"
                n772 = local read "rf step length 10"() -> (w848:dbl)
                n773 = local read "rf step length 9"() -> (w855:dbl)
                n774 = local read "rf step length 7"() -> (w852:dbl)
                n775 = local read "rf step length 8"() -> (w856:dbl)
                n776 = local read "rf step length 6"() -> (w851:dbl)
                n777 = local read "rf step length 4"() -> (w860:dbl)
                n778 = local read "rf step length 2"() -> (w863:dbl)
                n779 = local read "rf step length 3"() -> (w859:dbl)
                n780 = local read "rf step length 1"() -> (w864:dbl)
                n781 = local read "rf step length 5"() -> (w847:dbl)
                n782 = Number To Decimal String(number=w855) -> (decimal integer string=w812:string)  [unwired: 1 in]
                n783 = Number To Decimal String(number=w848) -> (decimal integer string=w814:string)  [unwired: 1 in]
                n784 = Number To Decimal String(number=w852) -> (decimal integer string=w808:string)  [unwired: 1 in]
                n785 = Number To Decimal String(number=w856) -> (decimal integer string=w810:string)  [unwired: 1 in]
                n786 = Number To Decimal String(number=w851) -> (decimal integer string=w806:string)  [unwired: 1 in]
                n787 = Number To Decimal String(number=w860) -> (decimal integer string=w818:string)  [unwired: 1 in]
                n788 = Number To Decimal String(number=w863) -> (decimal integer string=w822:string)  [unwired: 1 in]
                n789 = Number To Decimal String(number=w859) -> (decimal integer string=w820:string)  [unwired: 1 in]
                n790 = Number To Decimal String(number=w864) -> (decimal integer string=w824:string)  [unwired: 1 in]
                n791 = Number To Decimal String(number=w847) -> (decimal integer string=w816:string)  [unwired: 1 in]
                n792 = Concatenate Strings("RF Step 9 length" ("string"), w797, w797, w797, ":" ("string"), "\t", w812, "\r\n") -> (w837:string)
                n793 = Concatenate Strings("RF Step 10 length" ("string"), w800, w800, w800, ":" ("string"), "\t", w814, "\r\n") -> (w836:string)
                n794 = Concatenate Strings("RF Step 7 length" ("string"), w794, w794, w794, ":" ("string"), "\t", w808, "\r\n") -> (w839:string)
                n795 = Concatenate Strings("RF Step 8 length" ("string"), w795, w795, w795, ":" ("string"), "\t", w810, "\r\n") -> (w838:string)
                n796 = Concatenate Strings("RF Step 6 length" ("string"), w792, w792, w792, ":" ("string"), "\t", w806, "\r\n") -> (w840:string)
                n797 = Concatenate Strings("RF Step 4 length" ("string"), w787, w787, w787, ":" ("string"), "\t", w818, "\r\n") -> (w842:string)
                n798 = Concatenate Strings("RF Step 5 length" ("string"), w790, w790, w790, ":" ("string"), "\t", w816, "\r\n") -> (w841:string)
                n799 = Concatenate Strings("RF Step 2 length" ("string"), w783, w783, w783, ":" ("string"), "\t", w822, "\r\n") -> (w844:string)
                n800 = Concatenate Strings("RF Step 3 length" ("string"), w785, w785, w785, ":" ("string"), "\t", w820, "\r\n") -> (w843:string)
                n801 = Concatenate Strings("RF Step 1 length" ("string"), w782, w782, w782, ":" ("string"), "\t", w824, "\r\n") -> (w845:string)
                n802 = Concatenate Strings(w845, w844, w843, w842, w841) -> (w805:string)
                n803 = Concatenate Strings(w840, w839, w838, w837, w836) -> (w801:string)
                n804 = local read "Pressure set mbar"() -> (w763:dbl)
                n805 = local read "Step Number DC"() -> (w747:u16)
                n806 = local read "Step Number RF"() -> (w754:u16)
                n807 = local read "Ar set sccm"() -> (w774:dbl)
                n808 = Number To Decimal String(number=w747) -> (decimal integer string=w746:string)  [unwired: 1 in]
                n809 = Number To Decimal String(number=w774) -> (decimal integer string=w778:string)  [unwired: 1 in]
                n810 = Format Into String(format string="%.;%f", w763) -> (resulting string=w762:string)  [unwired: 2 in, 1 out]
                n811 = Number To Decimal String(number=w754) -> (decimal integer string=w753:string)  [unwired: 1 in]
                n812 = Concatenate Strings("Argon Flow(sccm)" ("string"), w779, w779, w779, ":" ("string"), "\t", w778, "\r\n") -> (w768:string)
                n813 = Concatenate Strings("Pressure(mbarr)" ("string"), w770, w770, w770, ":" ("string"), "\t", w762, "\r\n") -> (w766:string)
                n814 = Concatenate Strings("RF Step Number " ("string"), w760, w760, w760, ":" ("string"), "\t", w753, "\r\n") -> (w755:string)
                n815 = Concatenate Strings("DC Step Number" ("string"), w749, w749, w749, ":" ("string"), "\t", w746, "\r\n") -> (w745:string)
                n816 = Concatenate Strings(w756, w756, w755, w745) -> (w744:string)
                n817 = Concatenate Strings(w767, w767, w768, w766, w744) -> (w765:string)
                n818 = Concatenate Strings(w804, w804, w805, w801, w765) -> (w866:string)
                n819 = Concatenate Strings(w803, w866) -> (w802:string)
              }
              frame #6 {
                n820 = local read "Recipe Name"() -> (w872:string)
                n821 = call "File Dialog2"("start path"=path "D:/VK-1701 System Files/Recipe Files", "default name"=w872) -> ("selected path"=w870:path, "cancelled"=w869:bool, "error out"=→"error out":errorcluster)  [unwired: 10 in, 1 out]
                n822 = case shown="True" w869 {
                  tunnel: w870 -> [w882 _]
                  tunnel: [w882 path "" ("selected path")] -> w867
                  frame False {
                  }
                  frame True {
                  }
                }
                n823 = case shown="False" w869 {
                  tunnel: w868 -> [w875 _]
                  tunnel: w867 -> [w874 _]
                  frame False {
                    n824 = Open/Create/Replace File(file path (use dialog)=w874, operation (0:open)=T4."replace or create", access (0:read/write)=enum16{"read/write", "read-only", "write-only"}."read/write") -> (refnum out=w877:refnum<file>, error out=w876:errorcluster)  [unwired: 3 in, 1 out]
                    n825 = Write to Text File(file (use dialog)=w877, text=w875, error in=w876) -> (refnum out=w879:refnum<file>, error out=w878:errorcluster)  [unwired: 1 in, 1 out]
                    n826 = Close File(refnum=w879, error in=w878) -> ()  [unwired: 2 out]
                  }
                  frame True {
                  }
                }
                "concatenated string" <- w868
              }
              frame #7 {
              }
            }
          }
        }
        n827 = Equal?(x="flexmag", y="password") -> (x = y?=w337:bool)
        n828 = And(x=w337, y="password") -> (x .and. y?=w335:bool)
        n829 = case shown="True" w335 {
          frame False {
          }
          frame True {
            n830 = property on="hidden tab" class="TabCtl (strict)"("Visible"=TRUE) -> ()  [unwired: 2 in, 2 out]
            n831 = property on="concatenated string" class="Str"("Visible"=TRUE) -> ()  [unwired: 2 in, 2 out]
          }
        }
        n832 = local read "CANCEL"() -> (w341:bool)
        n833 = Or(x=w342, y=w341) -> (x .or. y?=w343:bool)
      }
      n834 = while {
        stop <- w24 stop-if-true
        n835 = Wait Until Next ms Multiple(millisecond multiple=u32 300) -> ()  [unwired: 1 out]
        n836 = case shown="True" "LOAD" {
          frame False {
          }
          frame True {
            n837 = stacked-sequence {
              frame #0 {
                n838 = call "File Dialog"("start path"=path "D:/VK-1701 System Files/Recipe Files") -> ("selected path"=w42:path, "cancelled"=w41:bool, "error out"=→"error out 2":errorcluster)  [unwired: 11 in, 1 out]
                n839 = case shown="False" w41 {
                  tunnel: [w203 string[][] [] ("all rows")] -> w201
                  tunnel: w42 -> [w202 _]
                  frame False {
                    n840 = call-poly <vilib>:"Read Delimited Spreadsheet.vi"("file path (dialog if empty)"=w202) -> ("all rows"=w203:string[][])  [unwired: 9 in, 5 out]
                  }
                  frame True {
                  }
                }
                n841 = Index Array(array=w201, index (row) #1=0 ("index (row)"), index (col) #1=4 ("index (row)"), index (row) #2=1 ("index (row)"), index (col) #2=4 ("index (row)"), index (row) #3=4 ("index (row)"), index (col) #3=4 ("index (row)"), index (row) #4=5 ("index (row)"), index (col) #4=4 ("index (row)"), index (row) #5=8 ("index (row)"), index (col) #5=4 ("index (row)"), index (row) #6=9 ("index (row)"), index (col) #6=4 ("index (row)"), index (row) #7=10 ("index (row)"), index (col) #7=4 ("index (row)"), index (row) #8=13 ("index (row)"), index (col) #8=4 ("index (row)"), index (row) #9=14 ("index (row)"), index (col) #9=4 ("index (row)"), index (row) #10=17 ("index (row)"), index (col) #10=4 ("index (row)"), index (row) #11=18 ("index (row)"), index (col) #11=4 ("index (row)"), index (row) #12=21 ("index (row)"), index (col) #12=4 ("index (row)"), index (row) #13=28 ("index (row)"), index (col) #13=4 ("index (row)"), index (row) #14=29 ("index (row)"), index (col) #14=4 ("index (row)"), index (row) #15=30 ("index (row)"), index (col) #15=4 ("index (row)"), index (row) #16=31 ("index (row)"), index (col) #16=4 ("index (row)"), index (row) #17=32 ("index (row)"), index (col) #17=4 ("index (row)"), index (row) #18=33 ("index (row)"), index (col) #18=4 ("index (row)"), index (row) #19=34 ("index (row)"), index (col) #19=4 ("index (row)"), index (row) #20=35 ("index (row)"), index (col) #20=4 ("index (row)"), index (row) #21=36 ("index (row)"), index (col) #21=4 ("index (row)"), index (row) #22=37 ("index (row)"), index (col) #22=4 ("index (row)"), index (row) #23=40 ("index (row)"), index (col) #23=4 ("index (row)"), index (row) #24=41 ("index (row)"), index (col) #24=4 ("index (row)"), index (row) #25=42 ("index (row)"), index (col) #25=4 ("index (row)"), index (row) #26=43 ("index (row)"), index (col) #26=4 ("index (row)"), index (row) #27=44 ("index (row)"), index (col) #27=4 ("index (row)"), index (row) #28=45 ("index (row)"), index (col) #28=4 ("index (row)"), index (row) #29=46 ("index (row)"), index (col) #29=4 ("index (row)"), index (row) #30=47 ("index (row)"), index (col) #30=4 ("index (row)"), index (row) #31=48 ("index (row)"), index (col) #31=4 ("index (row)"), index (row) #32=49 ("index (row)"), index (col) #32=4 ("index (row)"), index (row) #33=54 ("index (row)"), index (col) #33=4 ("index (row)"), index (row) #34=55 ("index (row)"), index (col) #34=4 ("index (row)"), index (row) #35=56 ("index (row)"), index (col) #35=4 ("index (row)"), index (row) #36=57 ("index (row)"), index (col) #36=4 ("index (row)"), index (row) #37=58 ("index (row)"), index (col) #37=4 ("index (row)"), index (row) #38=59 ("index (row)"), index (col) #38=4 ("index (row)"), index (row) #39=60 ("index (row)"), index (col) #39=4 ("index (row)"), index (row) #40=61 ("index (row)"), index (col) #40=4 ("index (row)"), index (row) #41=62 ("index (row)"), index (col) #41=4 ("index (row)"), index (row) #42=63 ("index (row)"), index (col) #42=4 ("index (row)"), index (row) #43=66 ("index (row)"), index (col) #43=4 ("index (row)"), index (row) #44=67 ("index (row)"), index (col) #44=4 ("index (row)"), index (row) #45=68 ("index (row)"), index (col) #45=4 ("index (row)"), index (row) #46=69 ("index (row)"), index (col) #46=4 ("index (row)"), index (row) #47=70 ("index (row)"), index (col) #47=4 ("index (row)"), index (row) #48=71 ("index (row)"), index (col) #48=4 ("index (row)"), index (row) #49=72 ("index (row)"), index (col) #49=4 ("index (row)"), index (row) #50=73 ("index (row)"), index (col) #50=4 ("index (row)"), index (row) #51=74 ("index (row)"), index (col) #51=4 ("index (row)"), index (row) #52=75 ("index (row)"), index (col) #52=4 ("index (row)"), index (row) #53=78 ("index (row)"), index (col) #53=4 ("index (row)"), index (row) #54=79 ("index (row)"), index (col) #54=4 ("index (row)"), index (row) #55=82 ("index (row)"), index (col) #55=4 ("index (row)"), index (row) #56=83 ("index (row)"), index (col) #56=4 ("index (row)")) -> (element #1=→"L recipe name":string, element #2=→"L sbs name":string, element #3=→"L recipe selection":string, element #4=→"L web selection":string, element #5=→"L core diamater":string, element #6=→"L left init diamater":string, element #7=→"L web thickness":string, element #8=→"L web speed":string, element #9=→"L tension  value":string, element #10=→"L single process type selection":string, element #11=→"L chamber selection":string, element #12=→"L microwave power":string, element #13=→"L dc power step 1":string, element #14=→"L dc power step 2":string, element #15=→"L dc power step 3":string, element #16=→"L dc power step 4":string, element #17=→"L dc power step 5":string, element #18=→"L dc power step 6":string, element #19=→"L dc power step 7":string, element #20=→"L dc power step 8":string, element #21=→"L dc power step 9":string, element #22=→"L dc power step 10":string, element #23=→"L dc length step 1":string, element #24=→"L dc length step 2":string, element #25=→"L dc length step 3":string, element #26=→"L dc length step 4":string, element #27=→"L dc length step 5":string, element #28=→"L dc length step 6":string, element #29=→"L dc length step 7":string, element #30=→"L dc length step 8":string, element #31=→"L dc length step 9":string, element #32=→"L dc length step 10":string, element #33=→"L rf power step 1":string, element #34=→"L rf power step 2":string, element #35=→"L rf power step 3":string, element #36=→"L rf power step 4":string, element #37=→"L rf power step 5":string, element #38=→"L rf power step 6":string, element #39=→"L rf power step 7":string, element #40=→"L rf power step 8":string, element #41=→"L rf power step 9":string, element #42=→"L rf power step 10":string, element #43=→"L rf length step 1":string, element #44=→"L rf length step 2":string, element #45=→"L rf length step 3":string, element #46=→"L rf length step 4":string, element #47=→"L rf length step 5":string, element #48=→"L rf length step 6":string, element #49=→"L rf length step 7":string, element #50=→"L rf length step 8":string, element #51=→"L rf length step 9":string, element #52=→"L rf length step 10":string, element #53=→"L argon flow":string, element #54=→"L pressure":string, element #55=→"L rf step number":string, element #56=→"L dc step number":string)
              }
              frame #1 {
                n842 = local read "L dc power step 10"() -> (w274:string)
                n843 = local read "L dc power step 9"() -> (w281:string)
                n844 = local read "L dc power step 8"() -> (w280:string)
                n845 = local read "L dc power step 1"() -> (w298:string)
                n846 = local read "L dc power step 7"() -> (w276:string)
                n847 = local read "L dc power step 2"() -> (w299:string)
                n848 = local read "L dc power step 4"() -> (w284:string)
                n849 = local read "L dc power step 3"() -> (w285:string)
                n850 = local read "L dc power step 5"() -> (w271:string)
                n851 = local read "L dc power step 6"() -> (w277:string)
                n852 = local read "L recipe selection"() -> (w319:string)
                n853 = local read "L web selection"() -> (w315:string)
                n854 = local read "L recipe name"() -> (w321:string)
                n855 = local read "L sbs name"() -> (w320:string)
                n856 = Decimal String To Number(string=w274) -> (number=w273:i32)  [unwired: 2 in, 1 out]
                n857 = Decimal String To Number(string=w281) -> (number=w282:i32)  [unwired: 2 in, 1 out]
                n858 = Decimal String To Number(string=w280) -> (number=w279:i32)  [unwired: 2 in, 1 out]
                n859 = Decimal String To Number(string=w298) -> (number=w297:i32)  [unwired: 2 in, 1 out]
                n860 = Decimal String To Number(string=w276) -> (number=w275:i32)  [unwired: 2 in, 1 out]
                n861 = Decimal String To Number(string=w299) -> (number=w300:i32)  [unwired: 2 in, 1 out]
                n862 = Decimal String To Number(string=w284) -> (number=w283:i32)  [unwired: 2 in, 1 out]
                n863 = Decimal String To Number(string=w285) -> (number=w286:i32)  [unwired: 2 in, 1 out]
                n864 = Decimal String To Number(string=w271) -> (number=w272:i32)  [unwired: 2 in, 1 out]
                n865 = Decimal String To Number(string=w277) -> (number=w278:i32)  [unwired: 2 in, 1 out]
                n866 = Equal?(x=w315, y="Web") -> (x = y?=w313:bool)
                n867 = Equal?(x=w319, y="Single Recipe") -> (x = y?=w317:bool)
                n868 = local write "dc step watt 10"(w273) -> ()
                n869 = local write "dc step watt 9"(w282) -> ()
                n870 = local write "dc step watt 1"(w297) -> ()
                n871 = local write "dc step watt 8"(w279) -> ()
                n872 = local write "dc step watt 7"(w275) -> ()
                n873 = local write "dc step watt 2"(w300) -> ()
                n874 = local write "dc step watt 4"(w283) -> ()
                n875 = local write "dc step watt 3"(w286) -> ()
                n876 = local write "dc step watt 5"(w272) -> ()
                n877 = local write "dc step watt 6"(w278) -> ()
                n878 = case shown="True" w317 {
                  tunnel: [w333 w334] -> w316
                  frame False {
                    w333 = u16 1 items=["single recipe", "multilayer recipe"] ("Recipe Selection")
                  }
                  frame True {
                    w334 = u16 0 items=["single recipe", "multilayer recipe"] ("Recipe Selection")
                  }
                }
                n879 = case shown="False" w313 {
                  tunnel: [w331 w332] -> w312
                  frame False {
                    w331 = u16 1 items=["web", "other"] ("Web Selection")
                  }
                  frame True {
                    w332 = u16 0 items=["web", "other"] ("Web Selection")
                  }
                }
                n880 = local write "Substrate Material"(w320) -> ()
                n881 = local write "Recipe Name"(w321) -> ()
                n882 = local read "L dc length step 1"() -> (w253:string)
                n883 = local read "L dc length step 10"() -> (w267:string)
                n884 = local read "L dc length step 7"() -> (w265:string)
                n885 = local read "L dc length step 2"() -> (w252:string)
                n886 = local read "L dc length step 4"() -> (w257:string)
                n887 = local read "L dc length step 9"() -> (w260:string)
                n888 = local read "L dc length step 3"() -> (w256:string)
                n889 = local read "L dc length step 5"() -> (w270:string)
                n890 = local read "L dc length step 6"() -> (w264:string)
                n891 = local read "L dc length step 8"() -> (w261:string)
                n892 = local write "Recipe Selection"(w316) -> ()
                n893 = local write "Web Selection"(w312) -> ()
                n894 = Wait (ms)(milliseconds to wait=u32 100) -> ()  [unwired: 1 out]
                n895 = Decimal String To Number(string=w253) -> (number=w254:i32)  [unwired: 2 in, 1 out]
                n896 = Decimal String To Number(string=w265) -> (number=w266:i32)  [unwired: 2 in, 1 out]
                n897 = Decimal String To Number(string=w252) -> (number=w251:i32)  [unwired: 2 in, 1 out]
                n898 = Decimal String To Number(string=w257) -> (number=w258:i32)  [unwired: 2 in, 1 out]
                n899 = Decimal String To Number(string=w260) -> (number=w259:i32)  [unwired: 2 in, 1 out]
                n900 = Decimal String To Number(string=w267) -> (number=w268:i32)  [unwired: 2 in, 1 out]
                n901 = Decimal String To Number(string=w256) -> (number=w255:i32)  [unwired: 2 in, 1 out]
                n902 = Decimal String To Number(string=w270) -> (number=w269:i32)  [unwired: 2 in, 1 out]
                n903 = Decimal String To Number(string=w264) -> (number=w263:i32)  [unwired: 2 in, 1 out]
                n904 = Decimal String To Number(string=w261) -> (number=w262:i32)  [unwired: 2 in, 1 out]
                n905 = local write "dc step length 1"(w254) -> ()
                n906 = local write "dc step length 10"(w268) -> ()
                n907 = local write "dc step length 7"(w266) -> ()
                n908 = local write "dc step length 2"(w251) -> ()
                n909 = local write "dc step length 4"(w258) -> ()
                n910 = local write "dc step length 9"(w259) -> ()
                n911 = local write "dc step length 3"(w255) -> ()
                n912 = local write "dc step length 5"(w269) -> ()
                n913 = local write "dc step length 6"(w263) -> ()
                n914 = local write "dc step length 8"(w262) -> ()
                n915 = local read "L microwave power"() -> (w295:string)
                n916 = local read "L left init diamater"() -> (w310:string)
                n917 = local read "L core diamater"() -> (w311:string)
                n918 = local read "L web thickness"() -> (w305:string)
                n919 = local read "L tension  value"() -> (w301:string)
                n920 = local read "L web speed"() -> (w304:string)
                n921 = Decimal String To Number(string=w295) -> (number=w296:i32)  [unwired: 2 in, 1 out]
                n922 = Decimal String To Number(string=w311) -> (number=w309:i32)  [unwired: 2 in, 1 out]
                n923 = Decimal String To Number(string=w305) -> (number=w306:i32)  [unwired: 2 in, 1 out]
                n924 = Decimal String To Number(string=w301) -> (number=w302:i32)  [unwired: 2 in, 1 out]
                n925 = Decimal String To Number(string=w304) -> (number=w303:i32)  [unwired: 2 in, 1 out]
                n926 = Fract/Exp String To Number(use system decimal point (T)=FALSE, string=w310) -> (number=w308:dbl)  [unwired: 2 in, 1 out]
                n927 = local write "power microwave"(w296) -> ()
                n928 = local write "left initial diameter"(w308) -> ()
                n929 = local write "core diameter"(w309) -> ()
                n930 = local write "web thickness"(w306) -> ()
                n931 = local write "tension value"(w302) -> ()
                n932 = local write "web speed"(w303) -> ()
                n933 = local read "L rf power step 10"() -> (w227:string)
                n934 = local read "L rf power step 9"() -> (w220:string)
                n935 = local read "L rf power step 8"() -> (w221:string)
                n936 = local read "L rf power step 1"() -> (w213:string)
                n937 = local read "L rf power step 7"() -> (w225:string)
                n938 = local read "L dc power step 6"() -> (w224:string)
                n939 = local read "L rf power step 2"() -> (w212:string)
                n940 = local read "L rf power step 4"() -> (w217:string)
                n941 = local read "L rf power step 3"() -> (w216:string)
                n942 = local read "L rf power step 5"() -> (w230:string)
                n943 = Decimal String To Number(string=w227) -> (number=w228:i32)  [unwired: 2 in, 1 out]
                n944 = local read "L single process type selection"() -> (w294:string)
                n945 = Decimal String To Number(string=w220) -> (number=w219:i32)  [unwired: 2 in, 1 out]
                n946 = Decimal String To Number(string=w221) -> (number=w222:i32)  [unwired: 2 in, 1 out]
                n947 = Decimal String To Number(string=w213) -> (number=w214:i32)  [unwired: 2 in, 1 out]
                n948 = Decimal String To Number(string=w225) -> (number=w226:i32)  [unwired: 2 in, 1 out]
                n949 = Decimal String To Number(string=w212) -> (number=w211:i32)  [unwired: 2 in, 1 out]
                n950 = Decimal String To Number(string=w217) -> (number=w218:i32)  [unwired: 2 in, 1 out]
                n951 = Decimal String To Number(string=w216) -> (number=w215:i32)  [unwired: 2 in, 1 out]
                n952 = Decimal String To Number(string=w230) -> (number=w229:i32)  [unwired: 2 in, 1 out]
                n953 = Decimal String To Number(string=w224) -> (number=w223:i32)  [unwired: 2 in, 1 out]
                n954 = local read "L chamber selection"() -> (w290:string)
                n955 = local write "rf step watt 10"(w228) -> ()
                n956 = local write "rf step watt 9"(w219) -> ()
                n957 = local write "rf step watt 8"(w222) -> ()
                n958 = local write "rf step watt 1"(w214) -> ()
                n959 = local write "rf step watt 7"(w226) -> ()
                n960 = local write "rf step watt 2"(w211) -> ()
                n961 = local write "rf step watt 4"(w218) -> ()
                n962 = local write "rf step watt 3"(w215) -> ()
                n963 = local write "rf step watt 5"(w229) -> ()
                n964 = local write "rf step watt 6"(w223) -> ()
                n965 = Equal?(x=w290, y="III" ("L single process")) -> (x = y?=w288:bool)
                n966 = Equal?(x=w294, y="Microwave" ("L single process")) -> (x = y?=w292:bool)
                n967 = case shown="True" w292 {
                  tunnel: [w324 enum32{"microwave", "dcsputter", "rfsputter"}."microwave" ("single process selection")] -> w291
                  frame False {
                    n968 = local read "L single process type selection"() -> (w326:string)
                    n969 = Equal?(x=w326, y="RF Sputter" ("L single process")) -> (x = y?=w325:bool)
                    n970 = case shown="False" w325 {
                      tunnel: [enum32{"microwave", "dcsputter", "rfsputter"}."dcsputter" ("single process selection") enum32{"microwave", "dcsputter", "rfsputter"}."rfsputter" ("single process selection")] -> w324
                      frame False {
                      }
                      frame True {
                      }
                    }
                  }
                  frame True {
                  }
                }
                n971 = case shown="False" w288 {
                  tunnel: [enum32{"chamber II", "chamber III"}."chamber II" ("DC Sputter Chamber Selection") enum32{"chamber II", "chamber III"}."chamber III" ("DC Sputter Chamber Selection")] -> w287
                  frame False {
                  }
                  frame True {
                  }
                }
                n972 = local read "L pressure"() -> (w207:string)
                n973 = local read "L rf length step 1"() -> (w248:string)
                n974 = local read "L rf length step 10"() -> (w234:string)
                n975 = local read "L argon flow"() -> (w205:string)
                n976 = local read "L rf length step 7"() -> (w236:string)
                n977 = local read "L rf length step 2"() -> (w249:string)
                n978 = local read "L rf length step 4"() -> (w244:string)
                n979 = local read "L rf length step 9"() -> (w241:string)
                n980 = local read "L rf length step 3"() -> (w245:string)
                n981 = local read "L rf length step 5"() -> (w231:string)
                n982 = local read "L rf length step 6"() -> (w237:string)
                n983 = local read "L rf length step 8"() -> (w240:string)
                n984 = Fract/Exp String To Number(use system decimal point (T)=FALSE, string=w207) -> (number=w208:dbl)  [unwired: 2 in, 1 out]
                n985 = Decimal String To Number(string=w205) -> (number=w206:i32)  [unwired: 2 in, 1 out]
                n986 = Decimal String To Number(string=w248) -> (number=w247:i32)  [unwired: 2 in, 1 out]
                n987 = Decimal String To Number(string=w236) -> (number=w235:i32)  [unwired: 2 in, 1 out]
                n988 = Decimal String To Number(string=w249) -> (number=w250:i32)  [unwired: 2 in, 1 out]
                n989 = Decimal String To Number(string=w244) -> (number=w243:i32)  [unwired: 2 in, 1 out]
                n990 = Decimal String To Number(string=w241) -> (number=w242:i32)  [unwired: 2 in, 1 out]
                n991 = Decimal String To Number(string=w234) -> (number=w233:i32)  [unwired: 2 in, 1 out]
                n992 = Decimal String To Number(string=w245) -> (number=w246:i32)  [unwired: 2 in, 1 out]
                n993 = Decimal String To Number(string=w231) -> (number=w232:i32)  [unwired: 2 in, 1 out]
                n994 = Decimal String To Number(string=w237) -> (number=w238:i32)  [unwired: 2 in, 1 out]
                n995 = Decimal String To Number(string=w240) -> (number=w239:i32)  [unwired: 2 in, 1 out]
                n996 = local write "DC Sputter Chamber Selection"(w287) -> ()
                n997 = local write "Pressure set mbar"(w208) -> ()
                n998 = local write "Ar set sccm"(w206) -> ()
                n999 = local write "rf step length 1"(w247) -> ()
                n1000 = local write "rf step length 10"(w233) -> ()
                n1001 = local write "rf step length 7"(w235) -> ()
                n1002 = local write "rf step length 2"(w250) -> ()
                n1003 = local write "rf step length 4"(w243) -> ()
                n1004 = local write "rf step length 9"(w242) -> ()
                n1005 = local write "rf step length 3"(w246) -> ()
                n1006 = local write "rf step length 5"(w232) -> ()
                n1007 = local write "rf step length 6"(w238) -> ()
                n1008 = local write "rf step length 8"(w239) -> ()
                n1009 = local write "single process selection"(w291) -> ()
              }
            }
          }
        }
        n1010 = local read "CANCEL"() -> (w26:bool)
        n1011 = local read "done"() -> (w25:bool)
        n1012 = Or(x=w25, y=w26) -> (x .or. y?=w24:bool)
      }
    }
  }
